vi "RT Main.vi"() -> ()   [LabVIEW 2018]
uses:
  <vilib>/rvi/interface/nirviOpenFPGA/nirviOpenFPGA.xnode
  <vilib>/rvi/interface/nirviMethod/nirviMethod.xnode
  <vilib>/FPGAPlugInAG/Dynamic/niLvFpga_Reset_Dynamic.vi
  <vilib>/FPGAPlugInAG/Dynamic/niLvFpga_Run_Dynamic.vi
  <vilib>/rvi/interface/nirviCloseFPGA/nirviCloseFPGA.xnode
  <vilib>/FPGAPlugInAG/Dynamic/niLvFpga_Close_Dynamic.vi
  <vilib>/FPGAPlugInAG/Dynamic/niLvFpga_Abort_Dynamic.vi
  <vilib>/rvi/interface/nirviReadWriteControl/nirviReadWriteControl.xnode
  NiFpgaLv.dll
  <vilib>/Utility/error.llb/Error Cluster From Error Code.vi
  <vilib>/rvi/interface/Simulation/niFpgaSimulationCallBeginRW.vi
  <vilib>/rvi/errors/niLvFpgaAdjustHostInterfaceError.vi
  <vilib>/ptbypt/NI_PtbyPt.lvlib
  <vilib>/addons/control/pid/NI_PID_pid.lvlib
  <vilib>/Analysis/NI_AALBase.lvlib
  <vilib>/Analysis/1siggen.llb/Ramp Pattern by Samples.vi
  FPGA Bitfiles/NVHLab_FPGATarget_MainFPGA_fVdYATQcYmw.lvbitx
  Main_FPGA.vi
  Controls/Output Range Brake.ctl
  Controls/Alarm1.ctl
  <vilib>/addons/control/pid/pid.llb/PID Output Rate Limiter (DBL).vi
  Controls/PID Gains.ctl
  Controls/Hydraulic1.ctl
  <vilib>/FPGAPlugInAG/cRIO-9082/niLvFpga_Open_cRIO-9082.vi
  <vilib>/rvi/interface/common/dynamic/niFpgaDynamicAddResources.vi
panel:
  out "Startwert Ramp H 2":dbl format="%#_3f"
  in  "stop 4":bool
  in  "stop 3":bool
  in  "stop 2":bool
  in  "Stop":bool
  in  "System Reset / ON":bool
  out "Alarms":T1
  in  "Alarme On":T2={"A 1"=TRUE, "A 2"=TRUE, "A 3"=TRUE, "A 4"=TRUE, "A 5"=TRUE, "A 6"=TRUE, "A 7"=TRUE, "A 8"=FALSE, "A 9"=TRUE, "A 10"=TRUE, "A 11"=TRUE, "A 12"=TRUE, "A 13"=TRUE, "A 14"=TRUE, "A 15"=TRUE, "A 16"=TRUE, "A 17"=TRUE, "A 18"=TRUE, "A 19"=TRUE, "A 20"=TRUE, "A 21"=TRUE, "A 22"=TRUE, "A 23"=TRUE, "A 24"=TRUE}
  in  "Master Alarm On":bool
  out "Master Alarm":bool
  in  "sample length LR":i32=100
  in  "sample length H":i32=100
  in  "Count (mSec) Normal LR":u32=10
  in  "Count (mSec) Ramp LR":u32=2
  in  "PID gains Brake L":T3={"proportional gain (Kc)"=0.3933188999071717, "integral gain (Kc*Ts/Ti)"=0.0018829701002687216, "derivative gain (Kc*Td/Ts)"=0.0} {"proportional gain (Kc)" format="%#_8g"; "integral gain (Kc*Ts/Ti)" format="%#_8g"}
  in  "PID gains Brake R":T3={"proportional gain (Kc)"=0.3933188999071717, "integral gain (Kc*Ts/Ti)"=0.0018829701002687216, "derivative gain (Kc*Td/Ts)"=0.0} {"proportional gain (Kc)" format="%#_8g"; "integral gain (Kc*Ts/Ti)" format="%#_8g"}
  in  "PID gains Brake H":T4={"proportional gain (Kc)"=5.0, "integral gain (Kc*Ts/Ti)"=0.1015625, "derivative gain (Kc*Td/Ts)"=0.0}
  in  "PID gains Speed Control":T4={"proportional gain (Kc)"=0.5, "integral gain (Kc*Ts/Ti)"=0.01171875, "derivative gain (Kc*Td/Ts)"=0.01171875}
  in  "sample length DM":i32=100
  in  "Count (mSec) Speed Control":u32=22
  in  "Count (mSec) H":u32=10
  in  "Output Range Brake R":T5={"Output high"=0.5, "Output low"=-0.5}
  in  "Output Range Brake L":T5={"Output high"=0.5, "Output low"=-0.5}
  in  "FeedFw_Ena":bool
  in  "Count (mSec) Ramp H":u32=2
  out "Mod6/Unit H":bool
  in  "output rate (EGU/min)":dbl=10000.0 format="%.2f"
  in  "Tq_Cal_H":cluster{"Gain_H":dbl, "Offset_H":dbl}={"Gain_H"=196.33, "Offset_H"=-10.8688} {"Offset_H" format="%#_13g"; "Gain_H" format="%#_13g"}
  in  "ACC_FeedFw":dbl
  in  "output range":T6={"output high"=10.0, "output low"=-3.0}
  in  "Speed_Ref_Cal_H":dbl
  in  "ESTOP":bool
  in  "Tq_Cal_L":cluster{"Gain":dbl, "Offset":dbl}={"Gain"=-175.0, "Offset"=-8.0} {"Offset" format="%#_13g"; "Gain" format="%#_13g"}
  in  "Tq_Cal_R":cluster{"Gain":dbl, "Offset":dbl}={"Gain"=-230.0, "Offset"=16.0} {"Offset" format="%#_13g"; "Gain" format="%#_13g"}
  in  "Spd_Cal_L":cluster{"Gain":dbl, "Offset":dbl}={"Gain"=298.85, "Offset"=0.0} {"Offset" format="%#_13g"; "Gain" format="%#_13g"}
  in  "Spd_Cal_R":cluster{"Gain":dbl, "Offset":dbl}={"Gain"=298.85, "Offset"=0.0} {"Offset" format="%#_13g"; "Gain" format="%#_13g"}
  in  "Spd_Cal_H":cluster{"Gain":dbl, "Offset":dbl}={"Gain"=800.0, "Offset"=100.0} {"Offset" format="%#_13g"; "Gain" format="%#_13g"}
  in  "milliseconds to wait Ramp LR":u32=10
  in  "type Ramp LR":u16(ring) items=["Linear", "Logarithmic"]
  out "Output Ramp LR":dbl format="%.2f"
  out "Output Speed Control":dbl
  in  "milliseconds to wait Speed Control":u32=10
  in  "type Speed Control":u16(ring) items=["Linear", "Logarithmic"]
  in  "milliseconds to wait Ramp H":u32=10
  in  "type Ramp H":u16(ring) items=["Linear", "Logarithmic"]
  out "Output Ramp H":dbl
  in  "Tab Control":enum32{"H", "L-R", "H-L-R", "System"}(tab)
  in  "Engine Speed/Torque H":bool
  in  "Torque Reference H":dbl(slide) scale=-1250.0..1250.0
  out "Torque with Transmission  H":dbl(knob) scale=-2000.0..2000.0
  out "Torque Back":dbl(knob) scale=-2000.0..2000.0
  out "Engine Speed Back":dbl(knob) scale=0.0..8000.0
  in  "Brake_H":bool
  in  "Direction H":bool=TRUE
  in  "Reset_H":bool
  in  "Control_H":bool
  in  "Speed_Ref_H":bool=TRUE caption="Torque_Ref_H"
  out "Report H":T7
  in  "Speed \nReferance H":dbl(slide) scale=0.0..8000.0
  out "Speed with Transmission H":dbl(knob) scale=0.0..12000.0
  in  "Transmisssion H":dbl=1.0
  in  "Start Ramp H":dbl=880.0
  in  "End Ramp H":dbl=4800.0
  in  "Time (Sec) Ramp H":i32=60
  out "Ramp H Activ":bool
  in  "Ramp H Stop":bool
  in  "Ramp H Down":bool
  in  "Ramp H Start":bool
  out "Ramp H  LED":bool
  out "Startwert Ramp H":dbl format="%#_3f"
  in  "Transmission with H":bool=TRUE
  out "Startwert Ramp LR":dbl format="%#_3f"
  out "Ramp LR  LED":bool
  in  "Transmission LR\nwith":bool=TRUE
  in  "Ramp LR Start":bool
  in  "Ramp LR Down":bool
  in  "Ramp LR Stop":bool
  out "Ramp LR active":bool
  in  "Time (Sec) Ramp LR":i32=60
  in  "End Ramp LR":dbl=4800.0
  in  "Start Ramp LR":dbl=880.0
  out "Speed_Diff":dbl(knob) scale=-30.0..30.0
  in  "Torque_Reference_LR":dbl(slide) caption="Torque \nReference" scale=-2000.0..2000.0
  in  "Engine Speed/moment LR":bool
  out "Torque with Transmission":dbl(knob) scale=-400.0..400.0
  out "Torque right":dbl(knob) scale=-2000.0..2000.0
  out "Torque left":dbl(knob) scale=-2000.0..2000.0
  out "Engine Speed right":dbl(knob) scale=0.0..3000.0
  out "Engine Speed left":dbl(knob) scale=0.0..3000.0
  in  "Brake_LR":bool
  in  "Direction\nBackwards":bool caption="Forward"
  in  "Reset_LR":bool
  in  "Control_LR":bool
  in  "Speed_Ref":bool=TRUE caption="Torque_Ref"
  out "Report L-R":T8
  in  "Speed_Reference_LR":dbl(slide) caption="Speed\n Reference" scale=0.0..3000.0
  out "Speed with Transmission":dbl(knob) scale=0.0..5000.0
  in  "Transmission LR":dbl=1.0
  out "L OUT":dbl
  out "R OUT":dbl
  in  "Loss Factor":dbl=1.0
  out "Speed With Trs HLR H 4":dbl caption="Torque With Transmission H"
  out "Speed With Trs HLR H 3":dbl caption="Speed With Transmission H"
  out "Speed With Trs HLR H 2":dbl caption="Torque With Transmission"
  out "Speed With Trs HLR H":dbl caption="Speed With Transmission"
  in  "Torque_Reference_LR 3":dbl(slide) caption="Torque \nReference H" scale=-2000.0..2000.0
  in  "Speed_Reference_LR 3":dbl(slide) caption="Speed\n Reference H" scale=0.0..3000.0
  in  "Torque_Reference_LR 2":dbl(slide) caption="Torque \nReference" scale=-2000.0..2000.0
  in  "Speed_Reference_LR 2":dbl(slide) caption="Speed\n Reference" scale=0.0..3000.0
  out "R OUT 2":dbl caption="R OUT"
  out "L OUT 2":dbl caption="L OUT"
  out "Speed_Diff 2":dbl(knob) scale=-30.0..30.0
  out "Engine Speed right HLR 2":dbl(knob) caption="Engine Speed Back" scale=0.0..3000.0
  out "Engine Speed right HLR":dbl(knob) caption="Engine Speed right" scale=0.0..3000.0
  out "Engine Speed left HLR":dbl(knob) caption="Engine Speed left" scale=0.0..3000.0
  in  "HLR LR Brake":T9={"Speed_Ref"=TRUE, "Control_HLR"=FALSE, "Reset_HLR"=FALSE, "Direction\nBackwards 2"=FALSE, "Brake_HLR"=FALSE} caption="HLR"
  in  "HLR H":T10={"Start Ramp H"=880.0, "End Ramp H"=4800.0, "Time (Sec) Ramp H"=60, "Ramp H Active"=FALSE, "Ramp H Stop"=FALSE, "Ramp H Down"=FALSE, "Ramp H Start"=FALSE, "Ramp H  LED 2"=FALSE, "Startwert Ramp H 2"=0.0} caption="H" {"Startwert Ramp H 2" format="%#_3f"}
  in  "HLR LR":T11={"H Time (Sec) Ramp LR"=60, "H Start Ramp LR"=880.0, "H End Ramp LR"=4800.0, "Startwert Ramp LR 2"=0.0, "H Ramp LR Start"=FALSE, "H Ramp LR Down"=FALSE, "H Ramp LR Stop"=FALSE, "Ramp LR  LED 2"=FALSE, "Ramp LR active"=FALSE, "Transmission LR\nwith"=TRUE} caption="LR" {"Startwert Ramp LR 2" format="%#_3f"}
  out "Report H-L-R":T12
  in  "Tab Control 2":enum32{"Petrol Engine", "Electric Engine"}(tab)
  in  "Mode_Section":u16(ring) items=["Idle", "N_Alfa", "N_T"]
  out "Ramp Cruise Control  LED":bool
  in  "Cruise Control Down":bool
  in  "Cruise Control Stop":bool
  out "Cruise Control Aktive":bool
  in  "Cruise Control Start":bool
  in  "PID Regler Speed Control\nWave Torque Reference":bool
  in  "Engine\nStart":bool
  in  "Pre Glow\nOn":bool
  in  "Ignition\nOn":bool
  in  "Fuel\nOn":bool
  out "Speed Control":u8(slide) scale=0.0..100.0
  in  "Speed Control Soll":dbl(slide) scale=0.0..100.0
  in  "Release Speed Control":bool
  in  "Clutch\nOpen":bool=TRUE
  out "Clutch":cluster{"Open":bool, "Closed":bool}
  in  "Time (Sec) Speed Control":i32=20
  in  "End Cruise Control":dbl=100.0
  in  "Start Cruise Control":dbl
  in  "Load Percent of Engine Speed":bool
  in  "Percent":dbl=0.5
  in  "Temperature Control \nRelease":bool
  in  "Temperature Control\nWait":bool
  in  "E-Acc_1":T13={"Gain"=1.0, "OffSet"=0.0}
  in  "E-Acc_2":T13={"Gain"=1.0, "OffSet"=0.0}
  out "High M":fxp<+/-,24,5> format="%#.2g"
  out "End Position \nDown M":bool
  out "End Position \nUp M":bool
  out "Up M":bool
  out "Down M":bool
  in  "Release High M":bool
  in  "Direction High M":bool
  in  "Release Engine Speed M":bool
  in  "Direction Engine Speed M":bool
  in  "Release Brake M":bool
  in  "Run Button":bool
  in  "Hydraulic Pump Control":dbl=11.0
  in  "Manual":bool
  in  "Up Button":bool
  in  "Down Button":bool
  in  "RPMK":dbl=300.0
  in  "Torque Engine":dbl
  in  "Hydraulic Clutch":dbl
  # "without"
  # "Left"
  # "Right"
  # "LR"
  # "without"
  # "Left"
  # "Right"
  # "H"
  # "System not Ready!"
  # "Closed"
  # "%"
  # "%"
  # "%"
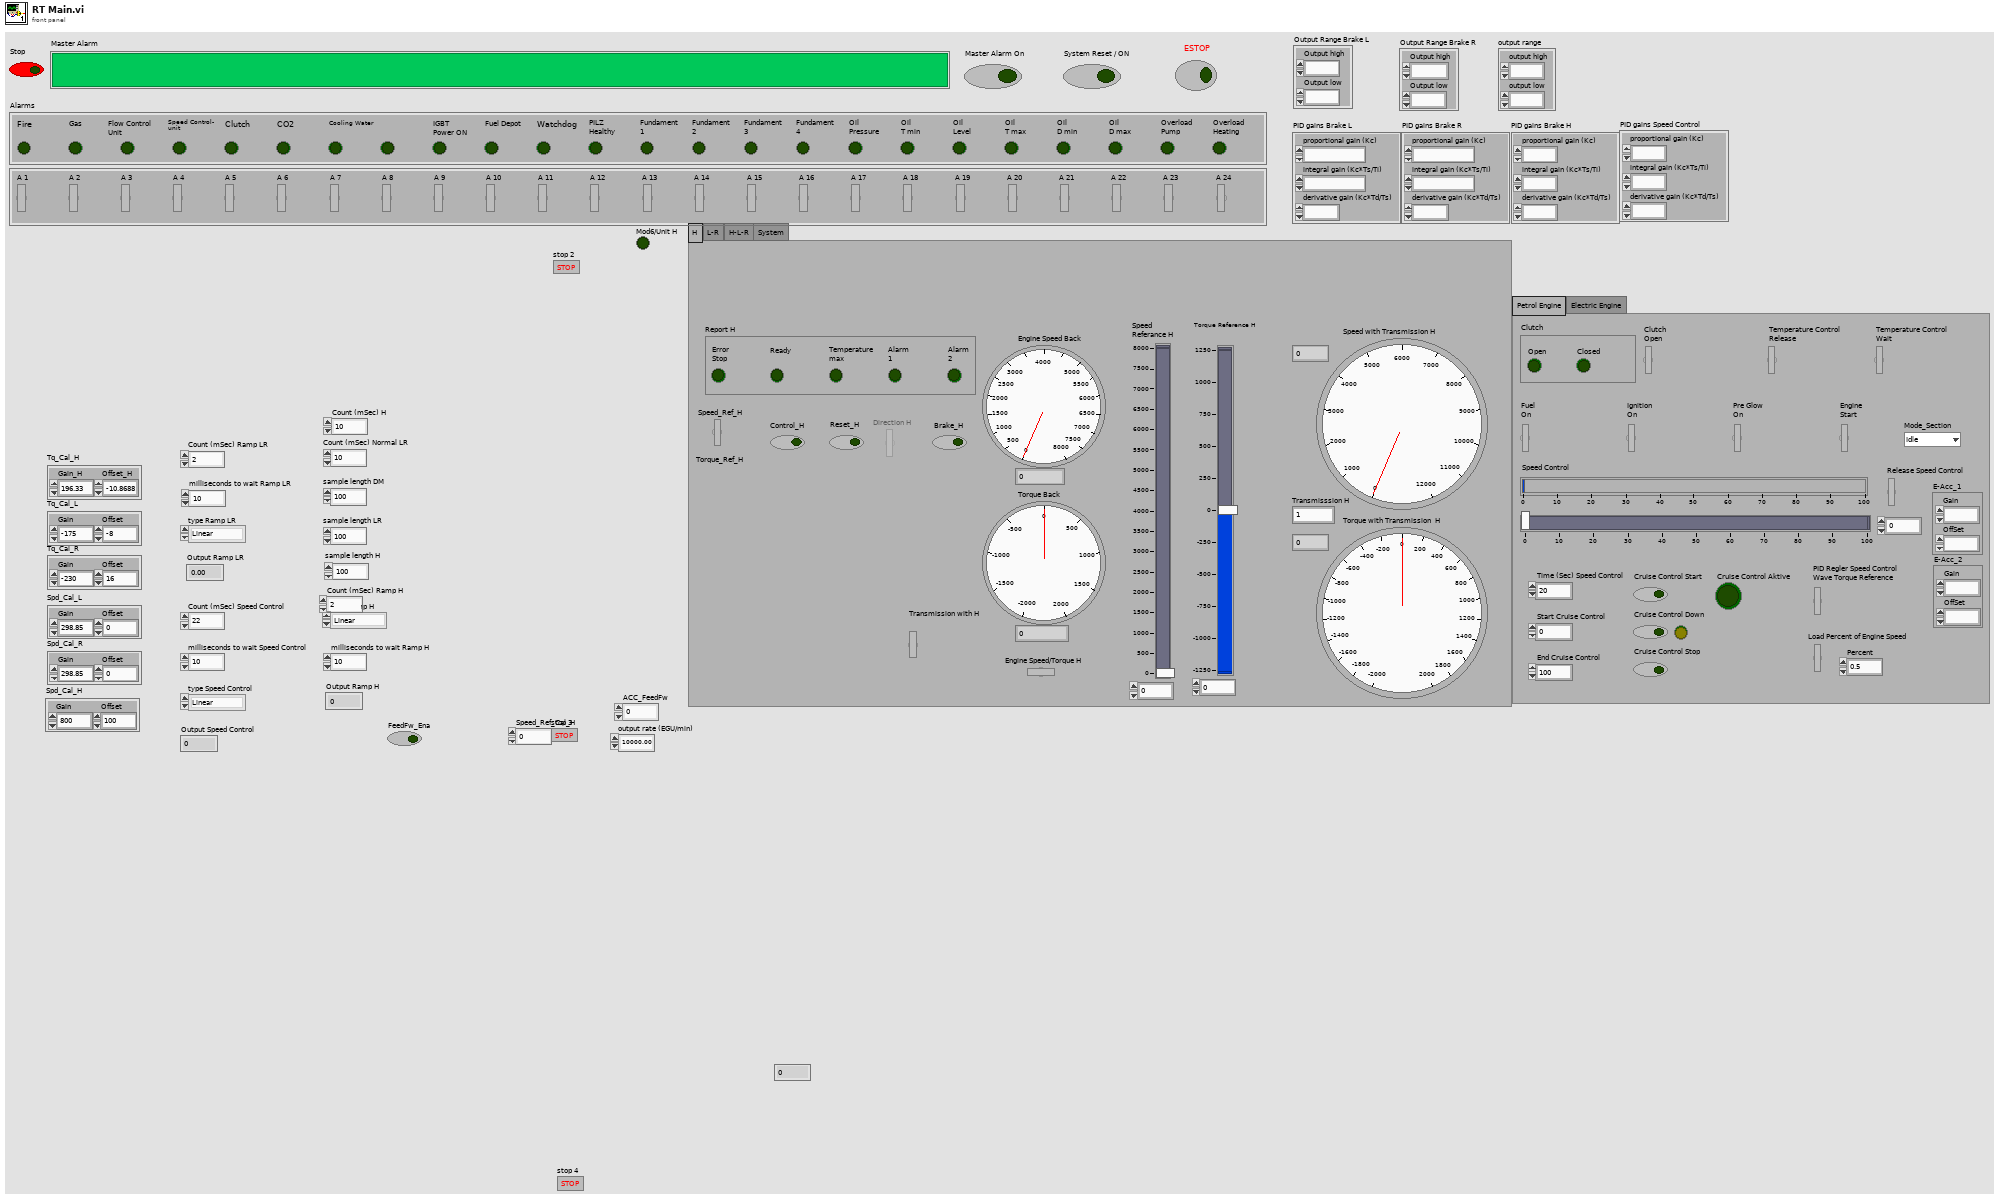
[diagram p1: front panel]
types:
  T1 = cluster{"Fire\n":bool, "Gas\n":bool, "Flow Control \nUnit":bool, "Speed Control-\nunit":bool, "Clutch\n":bool, "CO2\n":bool, "Cooling Water\n":bool, bool, "IGBT_ON":bool, "Fuel Depot\n":bool, "Watchdog\n":bool, "PILZ\nHealthy":bool, "Fundament\n1":bool, "Fundament\n2":bool, "Fundament\n3":bool, "Fundament\n4":bool, "Oil\nPressure":bool, "Oil\nT min":bool, "Oil\nLevel":bool, "Oil\nT max":bool, "Oil\nD min":bool, "Oil\nD max":bool, "Overload\nPump":bool, "Overload\nHeating":bool}
  T2 = typedef "Alarm1.ctl" = cluster{"A 1":bool, "A 2":bool, "A 3":bool, "A 4":bool, "A 5":bool, "A 6":bool, "A 7":bool, "A 8":bool, "A 9":bool, "A 10":bool, "A 11":bool, "A 12":bool, "A 13":bool, "A 14":bool, "A 15":bool, "A 16":bool, "A 17":bool, "A 18":bool, "A 19":bool, "A 20":bool, "A 21":bool, "A 22":bool, "A 23":bool, "A 24":bool}
  T3 = cluster{"proportional gain (Kc)":fxp<+/-,64,32>, "integral gain (Kc*Ts/Ti)":fxp<+/-,64,32>, "derivative gain (Kc*Td/Ts)":fxp<+/-,64,32>}
  T4 = cluster{"proportional gain (Kc)":fxp<+/-,16,8>, "integral gain (Kc*Ts/Ti)":fxp<+/-,16,8>, "derivative gain (Kc*Td/Ts)":fxp<+/-,16,8>}
  T5 = cluster{"Output high":fxp<+/-,64,32>, "Output low":fxp<+/-,64,32>}
  T6 = cluster{"output high":fxp<+/-,16,5>, "output low":fxp<+/-,16,5>}
  T7 = cluster{"Error\nStop":bool, "Ready\n":bool, "Temperature\nmax":bool, "Alarm\n1":bool, "Alarm\n2":bool}
  T8 = cluster{"Error\nStop":bool, "Ready\n":bool, "Temperature\nmax":bool, "Alarm\n1":bool, "Alarm\n2":bool, "Error\nStop":bool, "Ready\n":bool, "Temperature\nmax":bool, "Alarm\n1":bool, "Alarm\n2":bool}
  T9 = cluster{"Speed_Ref":bool, "Control_HLR":bool, "Reset_HLR":bool, "Direction\nBackwards 2":bool, "Brake_HLR":bool}
  T10 = cluster{"Start Ramp H":dbl, "End Ramp H":dbl, "Time (Sec) Ramp H":i32, "Ramp H Active":bool, "Ramp H Stop":bool, "Ramp H Down":bool, "Ramp H Start":bool, "Ramp H  LED 2":bool, "Startwert Ramp H 2":dbl}
  T11 = cluster{"H Time (Sec) Ramp LR":i32, "H Start Ramp LR":dbl, "H End Ramp LR":dbl, "Startwert Ramp LR 2":dbl, "H Ramp LR Start":bool, "H Ramp LR Down":bool, "H Ramp LR Stop":bool, "Ramp LR  LED 2":bool, "Ramp LR active":bool, "Transmission LR\nwith":bool}
  T12 = cluster{"Error\nStop":bool, "Ready\n":bool, "Temperature\nmax":bool, "Alarm\n1":bool, "Alarm\n2":bool, "Error\nStop":bool, "Ready\n":bool, "Temperature\nmax":bool, "Alarm\n1":bool, "Alarm\n2":bool, "H Error Stop\nStop 2":bool, "H Ready":bool, "H Temperature\nmax":bool, "H Alarm\n1":bool, "H Alarm2\n2":bool}
  T13 = cluster{"Gain":fxp<+/-,20,5>, "OffSet":fxp<+/-,20,5>}
  T14 = cluster{"Ramp Pattern":dbl[], "Ramp Type":u16, "Ramp Step":i32, "Ramp Start Cruise":dbl, "Ramp End  Cruise":dbl, "No of Ramps":i32, "Loop Time":u32, "LR Timer Done":bool, "LR Ramp On":bool, "Ramp Time Target":u32}
  T15 = cluster{"Ramp Pattern":dbl[], "Ramp Type":u16, "Ramp Step":i32, "Ramp Start H":dbl, "Ramp End  H":dbl, "No of Ramps":i32, "Loop Time":u32, "LR Timer Done":bool, "LR Ramp On":bool, "Ramp Time Target":u32}
  T16 = cluster{"FPGA VI Ref":refnum<k20>, "Ramp Pattern":dbl[], "Ramp Type":u16, "Ramp Step":i32, "Ramp Start LR":dbl, "Ramp End  LR":dbl, "No of Ramps":i32, "Loop Time":u32, "LR Timer Done":bool, "LR Ramp On":bool, "Ramp Time Target":u32}
  T17 = cluster{"System Reset / ON":bool, "Master Alarm On":bool, "Control_LR":bool, "Control_H":bool, "FeedFw_Ena":bool}
  T18 = typedef "Output Range Brake.ctl" = cluster{"Output Range Brake R":cluster{"Output high":fxp<+/-,64,32>, "Output low":fxp<+/-,64,32>}, "Output Range Brake L":cluster{"Output high":fxp<+/-,64,32>, "Output low":fxp<+/-,64,32>}, "output range":cluster{"output high":fxp<+/-,16,5>, "output low":fxp<+/-,16,5>}}
  T19 = typedef "PID Gains.ctl" = cluster{"PID gains Brake L":cluster{"proportional gain (Kc)":fxp<+/-,64,32>, "integral gain (Kc*Ts/Ti)":fxp<+/-,64,32>, "derivative gain (Kc*Td/Ts)":fxp<+/-,64,32>}, "PID gains Brake R":cluster{"proportional gain (Kc)":fxp<+/-,64,32>, "integral gain (Kc*Ts/Ti)":fxp<+/-,64,32>, "derivative gain (Kc*Td/Ts)":fxp<+/-,64,32>}, "PID gains Brake H":cluster{"proportional gain (Kc)":fxp<+/-,16,8>, "integral gain (Kc*Ts/Ti)":fxp<+/-,16,8>, "derivative gain (Kc*Td/Ts)":fxp<+/-,16,8>}, "PID gains Speed Control":cluster{"proportional gain (Kc)":fxp<+/-,16,8>, "integral gain (Kc*Ts/Ti)":fxp<+/-,16,8>, "derivative gain (Kc*Td/Ts)":fxp<+/-,16,8>}}
  T20 = typedef "Hydraulic1.ctl" = cluster{"Hydraulic Pump Control":dbl, "RPMK":dbl, "Down Button":bool, "Torque Engine":dbl, "Hydraulic Clutch":dbl, "Run Button":bool, "Up Button":bool}
  T21 = cluster{"Mod5/Alarm 1 Fire":bool, "Mod5/Alarm 2 Gas":bool, "Mod5/Alarm 3 Flow Control Unit":bool, "Mod5/Alarm 4 Speed Control":bool, "Mod5/Alarm 5 Clutch":bool, "Mod5/Alarm 6 CO2":bool, "Mod5/Alarm 7 Exhaust":bool, "Mod5/Alarm 8 Cooling Water":bool, "Mod5/Alarm 9 IGBT_ON":bool, "Mod5/Alarm 10 Fuel Depot":bool, "Mod5/Alarm 11 Watchdog":bool, "Mod5/Alarm 12 Spring Element":bool, "Mod5/Alarm 13 Fundament 1":bool, "Mod5/Alarm 14 Fundament 2":bool, "Mod5/Alarm 15 Fundament 3":bool, "Mod5/Alarm 16 Fundament 4":bool, "Mod6/Alarm 17 Oil Pressure Difference":bool, "Mod6/Alarm 19 min Oil Pressure":bool, "Mod6/Alarm 18 Oil Level":bool, "Mod6/Alarm 20 max Oil Temperature":bool, "Mod6/Alarm 21 min Oil Pressure":bool, "Mod6/Alarm 22 max Oil Pressure":bool, "Mod6/Alarm 23 Overload Warning Oil Pump":bool, "Mod6/Alarm 24 Overload Warning Oil Heating":bool}
  T22 = cluster{"Mod5/Error Brake L":bool, "Mod5/Ready Brake L":bool, "Mod5/Temperature Brake L":bool, "Mod5/Alarm 1 Brake L":bool, "Mod5/Alarm 2 Brake L":bool, "Mod5/Error Brake R":bool, "Mod5/Ready Brake R":bool, "Mod5/Temperature Brake R":bool, "Mod5/Alarm 1 Brake R":bool, "Mod5/Alarm 2 Brake R":bool}
  T23 = cluster{"Mod6/Error Brake back":bool, "Mod6/Ready Brake back":bool, "Mod6/Temperature Brake back":bool, "Mod6/Alarm 1 Brake back":bool, "Mod6/Alarm 2 Brake back":bool}
  T24 = cluster{"Mod6/Clutch open":bool, "Mod6/Clutch closed":bool}
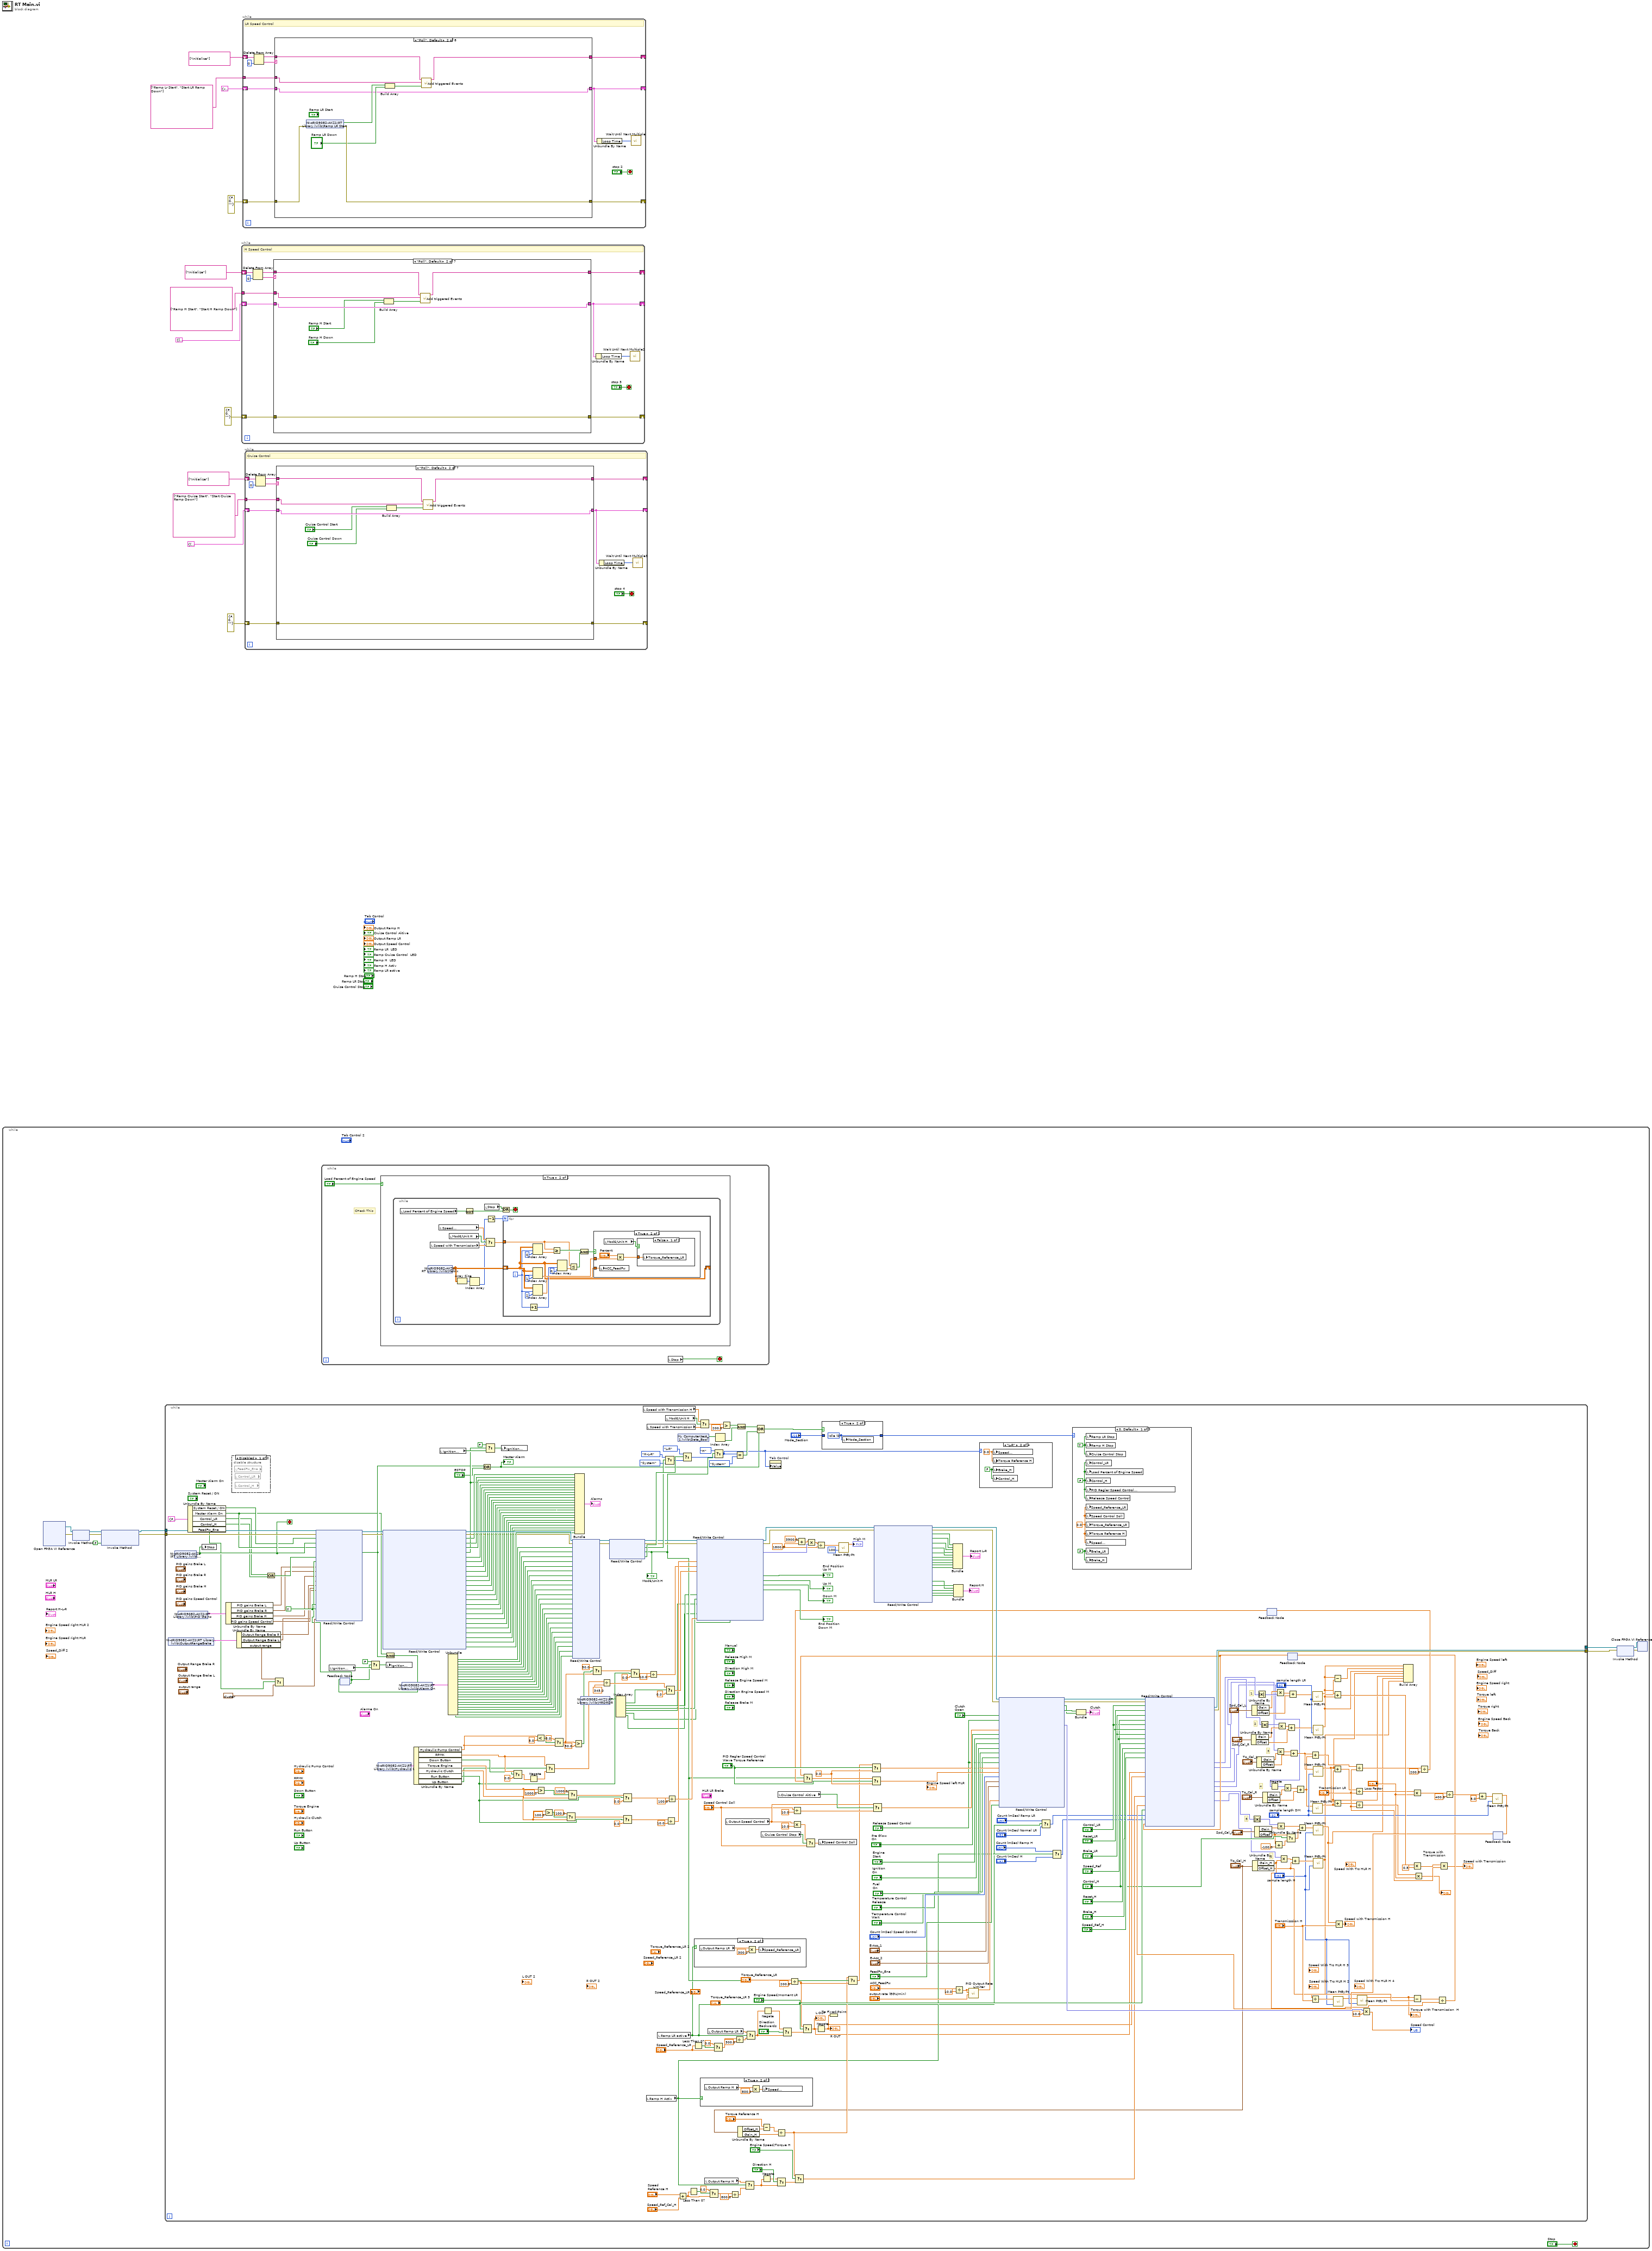
[diagram p0: block diagram]
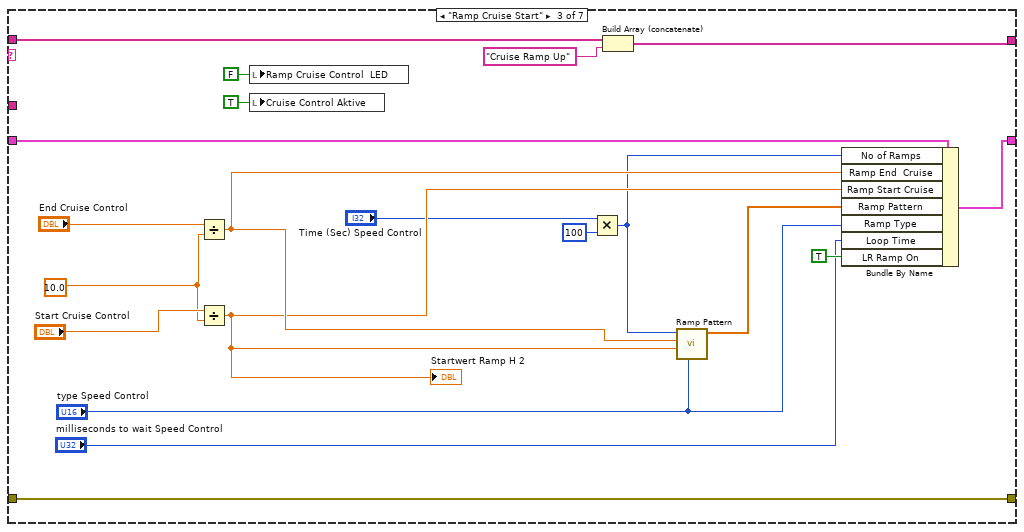
[diagram p3: hidden frame]
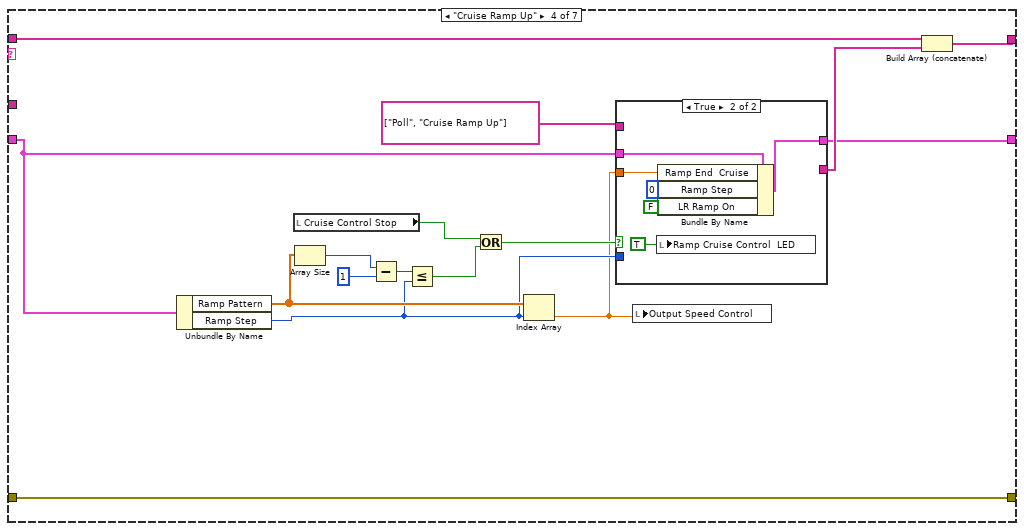
[diagram p4: hidden frame]
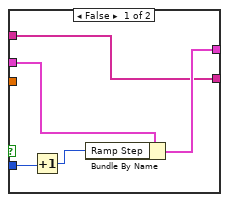
[diagram p5: hidden frame]
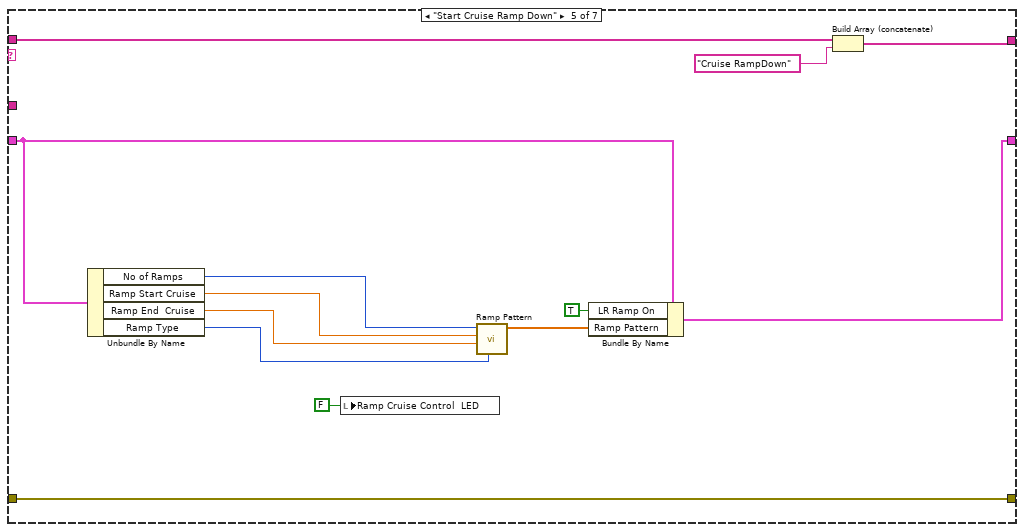
[diagram p6: hidden frame]
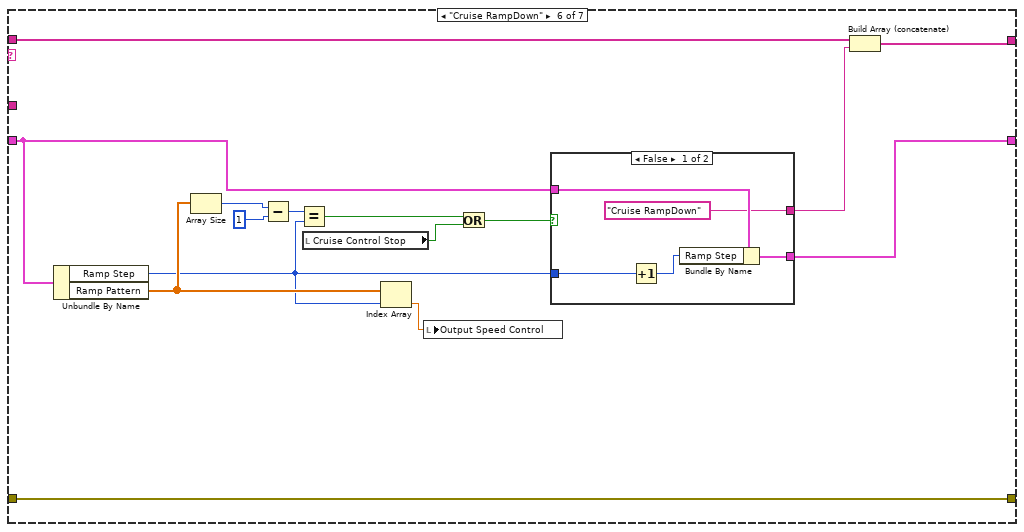
[diagram p7: hidden frame]
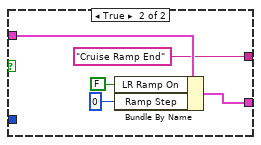
[diagram p8: hidden frame]
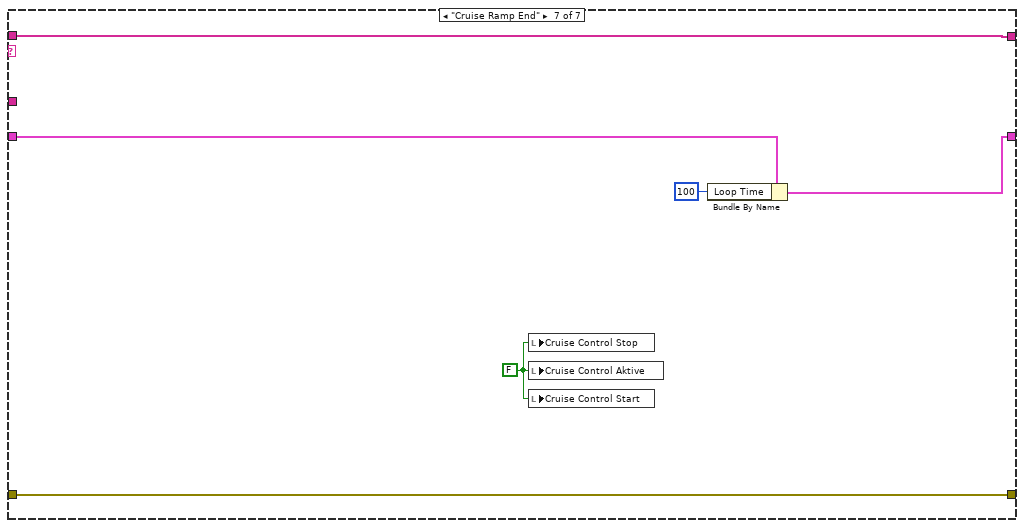
[diagram p9: hidden frame]
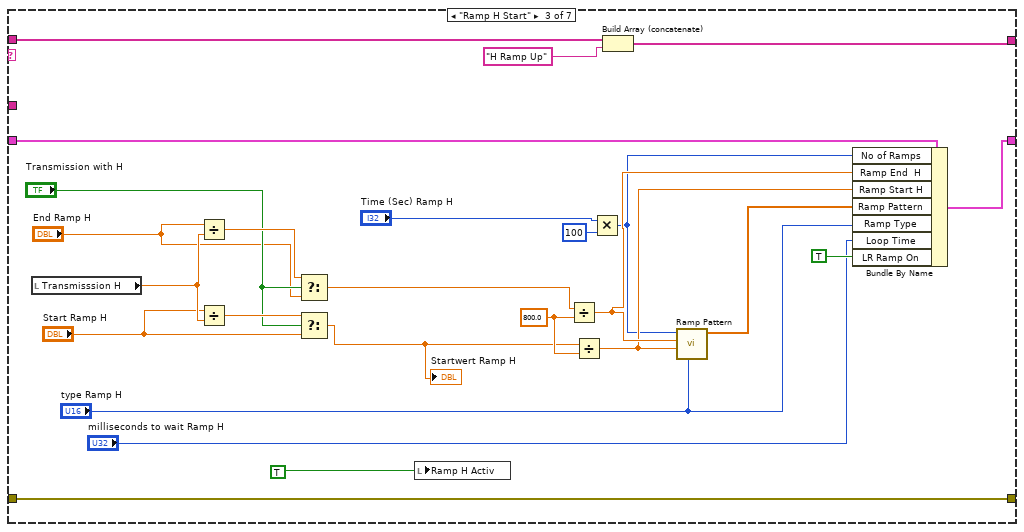
[diagram p11: hidden frame]
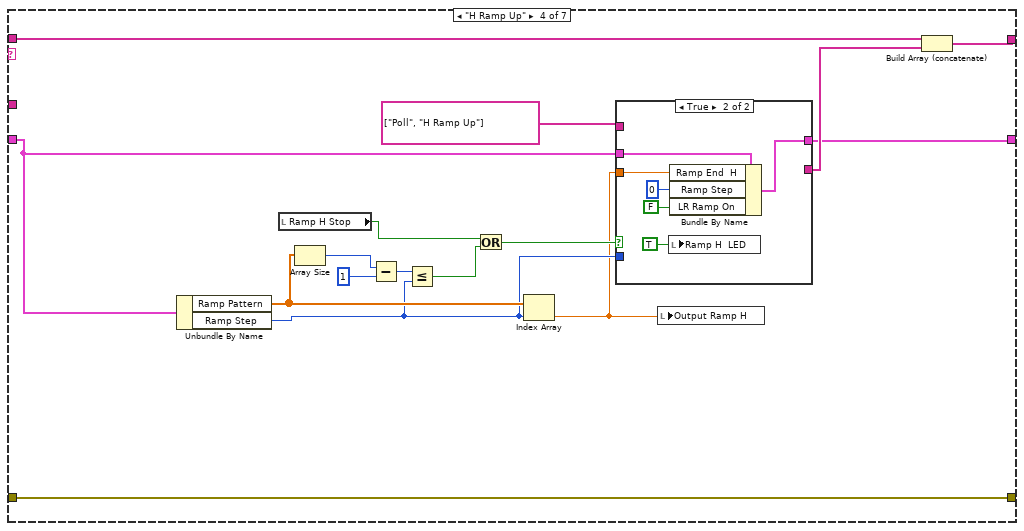
[diagram p12: hidden frame]
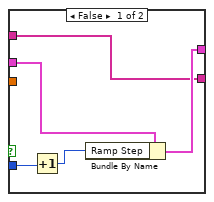
[diagram p13: hidden frame]
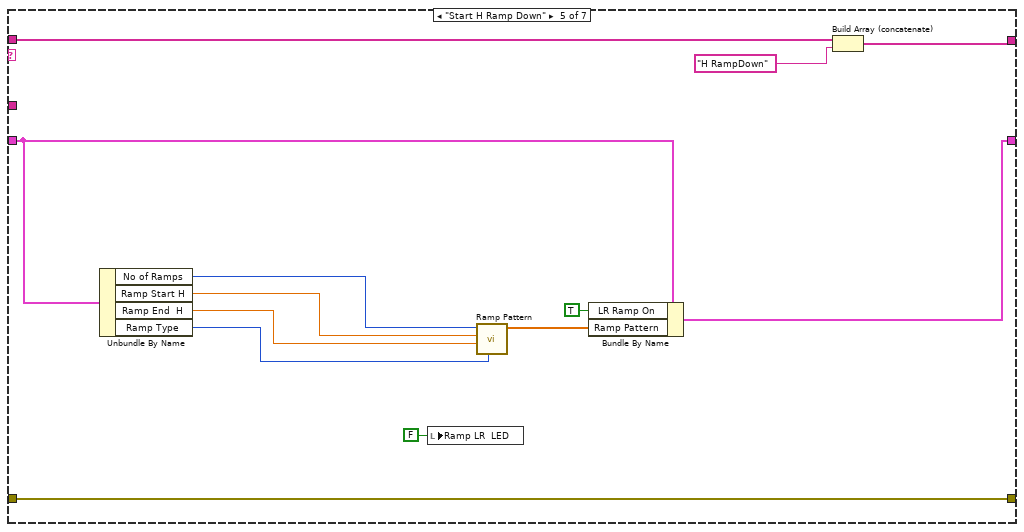
[diagram p14: hidden frame]
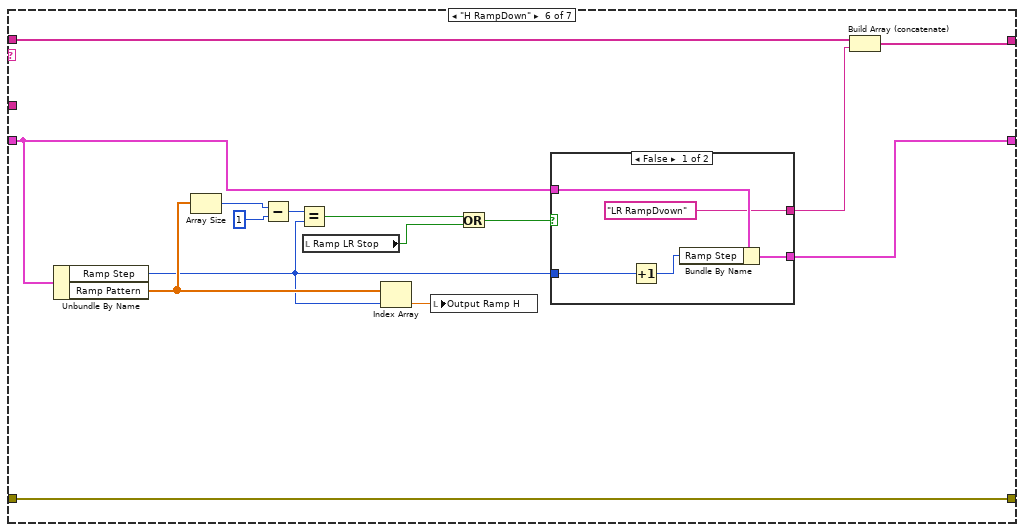
[diagram p15: hidden frame]
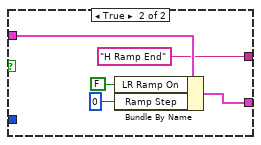
[diagram p16: hidden frame]
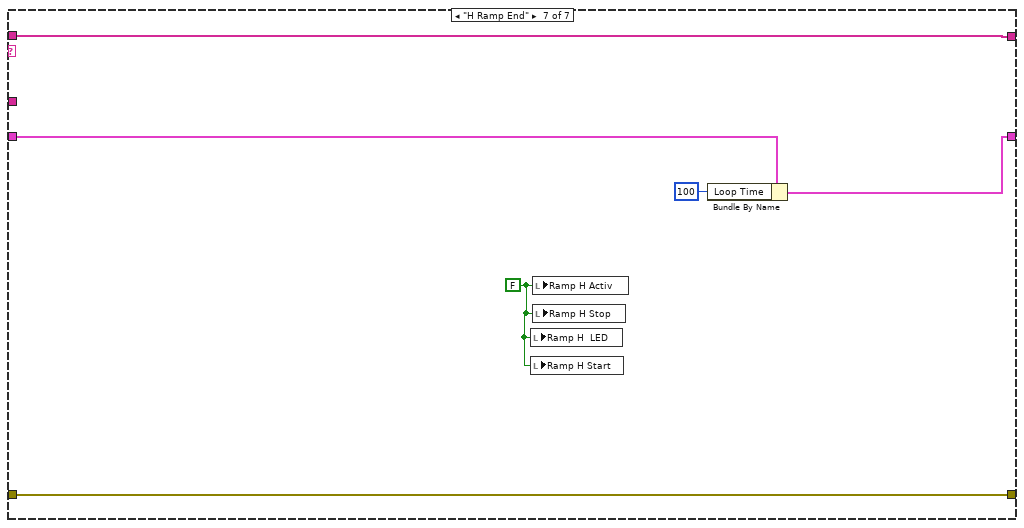
[diagram p17: hidden frame]
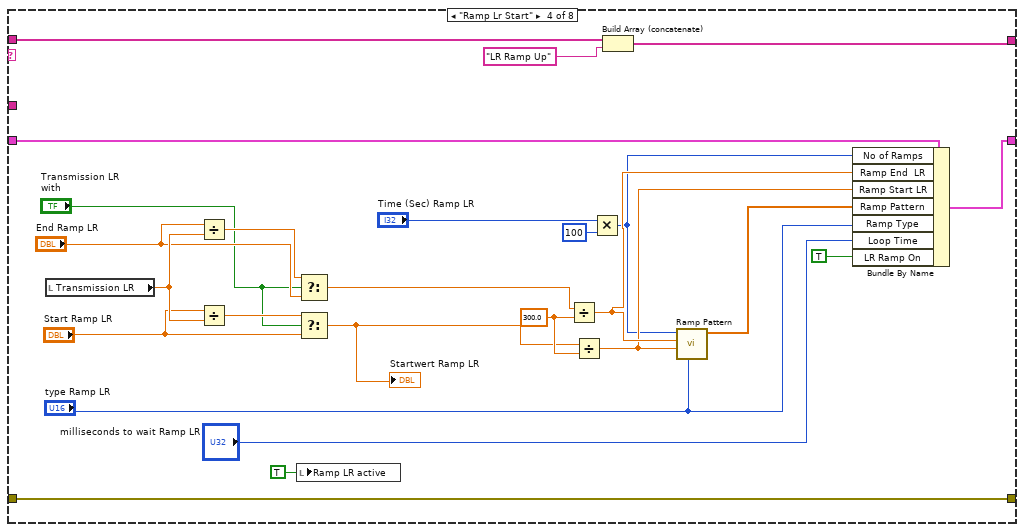
[diagram p20: hidden frame]
diagram:
  n1 = while {
    stop <- "Stop" stop-if-true
    n2 = xnode "Open FPGA VI Reference"() -> ("FPGA VI Reference Out"=w20:refnum<k20>, "error out"=w19:errorcluster)  [unwired: 2 in]
    n3 = xnode "Invoke Method"("FPGA VI Reference In"=w20, "error in"=w19) -> ("FPGA VI Reference Out"=w18:refnum<k20>, "error out"=w17:errorcluster)
    n4 = xnode "Invoke Method"("FPGA VI Reference In"=w18, "error in"=w17, "Wait Until Done (F)"=FALSE) -> ("FPGA VI Reference Out"=w13:refnum<k20>, "error out"=w24:errorcluster)
    n5 = while {
      tunnel: w13 -> [w439]
      tunnel: w24 -> [w438]
      tunnel: [w279] -> w23
      tunnel: [w308] -> w21
      stop <- w85 stop-if-true
      w220 = TRUE
      w261 = 0.0 ("f")
      w344 = 1800.0 ("y")
      # "6"
      # "5"
      # "4"
      # "3"
      # "2"
      # "1"
      n6 = shared-variable "NI-cRIO9082-AKZ1\\RT Library.lvlib\\OutputRangeBrake"() -> (w81:T18)  [unwired: 1 in, 1 out]
      n7 = shared-variable "NI-cRIO9082-AKZ1\\RT Library.lvlib\\Stop"() -> (w85:bool)  [unwired: 1 in, 1 out]
      n8 = shared-variable "NI-cRIO9082-AKZ1\\RT Library.lvlib\\PID Gains"() -> (w86:T19)  [unwired: 1 in, 1 out]
      n9 = Unbundle By Name(T17 {"System Reset / ON"=FALSE, "Master Alarm On"=FALSE, "Control_LR"=FALSE, "Control_H"=FALSE, "FeedFw_Ena"=FALSE}) -> ("System Reset / ON"=w79:bool, "Master Alarm On"=w78:bool, "Control_LR"=w77:bool, "Control_H"=w76:bool, "FeedFw_Ena"=w75:bool)
      n10 = local write "Stop"(w85) -> ()
      n11 = Unbundle By Name(w86) -> ("PID gains Brake L"=w90:T3, "PID gains Brake R"=w89:T3, "PID gains Brake H"=w88:T4, "PID gains Speed Control"=w87:T4)
      n12 = disable-structure shown="Disabled" {
        frame Disabled {
          n13 = local read "FeedFw_Ena"() -> ()  [unwired: 1 out]
          n14 = local read "Control_LR"() -> ()  [unwired: 1 out]
          n15 = local read "Control_H"() -> ()  [unwired: 1 out]
        }
        frame Enabled {
        }
      }
      n16 = Unbundle By Name(w81) -> ("Output Range Brake R"=w84:T5, "Output Range Brake L"=w83:T5, "output range"=w82:T6)
      n17 = Or(x=w77, y=w76) -> (x .or. y?=w288:bool)
      n18 = Select(t=w82, s=w75, f=T6 {"output high"=10.0, "output low"=0.0} ("output range")) -> (s? t:f=w176:T6)
      n19 = local read "Ignition\nOn"() -> (w238:bool)
      n20 = feedback #1() -> (w151:bool)  [unwired: 1 in]
      n21 = xnode "Read/Write Control"("FPGA VI Reference In"=w439, "error in"=w438, "Mod3/System Reset/ON"=w79, "STOP"=w85, "Alarm ON"=w78, "Mod3/Flashing light"=w288, "Mod3/Horn"=w151, "PID gains Brake L"=w90, "PID gains Brake R"=w89, "PID gains Brake H"=w88, "PID gains"=w87, "Output Range Brake R"=w84, "Output Range Brake L"=w83, "PID Out LR"=w220, "PID Out H"=w220, "output range"=w176) -> ("FPGA VI Reference Out"=w437:refnum<k20>, "error out"=w353:errorcluster, "Alarm"=w150:bool)  [unwired: 3 out]
      n22 = Select(t=FALSE, s=w151, f=w238) -> (s? t:f=w240:bool)
      n23 = shared-variable "NI-cRIO9082-AKZ1\\RT Library.lvlib\\Hydraulic 1"() -> (w92:T20)  [unwired: 1 in, 1 out]
      n24 = xnode "Read/Write Control"("FPGA VI Reference In"=w437, "error in"=w353) -> ("FPGA VI Reference Out"=w436:refnum<k20>, "error out"=w314:errorcluster, "Mod5/Alarm 1 Fire"=w435:bool, "Mod5/Alarm 2 Gas"=w434:bool, "Mod5/Alarm 3 Flow Control Unit"=w432:bool, "Mod5/Alarm 4 Speed Control"=w232:bool, "Mod5/Alarm 5 Clutch"=w431:bool, "Mod5/Alarm 6 CO2"=w430:bool, "Mod5/Alarm 7 Exhaust"=w215:bool, "Mod5/Alarm 8 Cooling Water"=w429:bool, "Mod5/Alarm 9 IGBT_ON"=w428:bool, "Mod5/Alarm 10 Fuel Depot"=w427:bool, "Mod5/Alarm 11 Watchdog"=w426:bool, "Mod5/Alarm 12 Spring Element"=w425:bool, "Mod5/Alarm 13 Fundament 1"=w424:bool, "Mod5/Alarm 14 Fundament 2"=w423:bool, "Mod5/Alarm 15 Fundament 3"=w422:bool, "Mod5/Alarm 16 Fundament 4"=w421:bool, "Mod6/Alarm 17 Oil Pressure Difference"=w420:bool, "Mod6/Alarm 19 min Oil Pressure"=w419:bool, "Mod6/Alarm 18 Oil Level"=w418:bool, "Mod6/Alarm 20 max Oil Temperature"=w417:bool, "Mod6/Alarm 21 min Oil Pressure"=w416:bool, "Mod6/Alarm 22 max Oil Pressure"=w415:bool, "Mod6/Alarm 23 Overload Warning Oil Pump"=w414:bool, "Mod6/Alarm 24 Overload Warning Oil Heating"=w413:bool)
      n25 = And(x=w78, y=w150) -> (x .and. y?=w363:bool)
      n26 = feedback-in #1(w363) -> ()
      n27 = local write "Ignition\nOn"(w240) -> ()
      n28 = shared-variable "NI-cRIO9082-AKZ1\\RT Library.lvlib\\Alarm On"() -> (w91:T2)  [unwired: 1 in, 1 out]
      n29 = Unbundle By Name(w92) -> ("Hydraulic Pump Control"=w99:dbl, "RPMK"=w98:dbl, "Down Button"=w97:bool, "Torque Engine"=w96:dbl, "Hydraulic Clutch"=w95:dbl, "Run Button"=w94:bool, "Up Button"=w93:bool)
      n30 = local read "Ignition\nOn"() -> (w235:bool)
      n31 = Unbundle(w91) -> ("A 1"=w411:bool, "A 2"=w410:bool, "A 3"=w409:bool, "A 4"=w408:bool, "A 5"=w407:bool, "A 6"=w406:bool, "A 7"=w405:bool, "A 8"=w404:bool, "A 9"=w403:bool, "A 10"=w402:bool, "A 11"=w401:bool, "A 12"=w400:bool, "A 13"=w399:bool, "A 14"=w398:bool, "A 15"=w397:bool, "A 16"=w396:bool, "A 17"=w395:bool, "A 18"=w394:bool, "A 19"=w393:bool, "A 20"=w392:bool, "A 21"=w391:bool, "A 22"=w390:bool, "A 23"=w389:bool, "A 24"=w388:bool)
      n32 = Or(x=w150, y="ESTOP") -> (x .or. y?=w149:bool)
      "Master Alarm" <- w149
      n33 = Select(t=FALSE, s=w232, f=w235) -> (s? t:f=w233:bool)
      n34 = local write "Ignition\nOn"(w233) -> ()
      n35 = Select(t=w98, s=w97, f=0.0) -> (s? t:f=w338:dbl)
      n36 = Negate(x=w338) -> (-x=w337:dbl)
      n37 = Less?(x=w99, y=5.0) -> (x < y?=w276:bool)
      n38 = Greater?(x=w96, y=1000.0) -> (0:w321:bool)
      n39 = Greater?(x=w95, y=100.0) -> (0:w285:bool)
      n40 = Select(t=w98, s=w93, f=w337) -> (s? t:f=w336:dbl)
      n41 = Select(t=5.0, s=w276, f=w99) -> (s? t:f=w274:dbl)
      n42 = Select(t=100.0, s=w285, f=w95) -> (s? t:f=w283:dbl)
      n43 = Select(t=1000.0, s=w321, f=w96) -> (s? t:f=w318:dbl)
      n44 = xnode "Read/Write Control"("FPGA VI Reference In"=w436, "error in"=w314, "Alarm 1 ON"=w411, "Alarm 2 ON"=w410, "Alarm 3 ON"=w409, "Alarm 4 ON"=w408, "Alarm 5 ON"=w407, "Alarm 6 ON"=w406, "Alarm 7 ON"=w405, "Alarm 8 ON"=w404, "Alarm 9 ON"=w403, "Alarm 10 ON"=w402, "Alarm 11 ON"=w401, "Alarm 12 ON"=w400, "Alarm 13 ON"=w399, "Alarm 14 ON"=w398, "Alarm 15 ON"=w397, "Alarm 16 ON"=w396, "Alarm 17 ON"=w395, "Alarm 18 ON"=w394, "Alarm 19 ON"=w393, "Alarm 20 ON"=w392, "Alarm 21 ON"=w391, "Alarm 22 ON"=w390, "Alarm 23 ON"=w389, "Alarm 24 ON"=w388) -> ("FPGA VI Reference Out"=w412:refnum<k20>, "error out"=w313:errorcluster)
      n45 = Greater?(x=w274, y=50.0) -> (0:w331:bool)
      n46 = Bundle("Mod5/Alarm 1 Fire"=w435, "Mod5/Alarm 2 Gas"=w434, "Mod5/Alarm 3 Flow Control Unit"=w432, "Mod5/Alarm 4 Speed Control"=w232, "Mod5/Alarm 5 Clutch"=w431, "Mod5/Alarm 6 CO2"=w430, "Mod5/Alarm 7 Exhaust"=w215, "Mod5/Alarm 8 Cooling Water"=w429, "Mod5/Alarm 9 IGBT_ON"=w428, "Mod5/Alarm 10 Fuel Depot"=w427, "Mod5/Alarm 11 Watchdog"=w426, "Mod5/Alarm 12 Spring Element"=w425, "Mod5/Alarm 13 Fundament 1"=w424, "Mod5/Alarm 14 Fundament 2"=w423, "Mod5/Alarm 15 Fundament 3"=w422, "Mod5/Alarm 16 Fundament 4"=w421, "Mod6/Alarm 17 Oil Pressure Difference"=w420, "Mod6/Alarm 19 min Oil Pressure"=w419, "Mod6/Alarm 18 Oil Level"=w418, "Mod6/Alarm 20 max Oil Temperature"=w417, "Mod6/Alarm 21 min Oil Pressure"=w416, "Mod6/Alarm 22 max Oil Pressure"=w415, "Mod6/Alarm 23 Overload Warning Oil Pump"=w414, "Mod6/Alarm 24 Overload Warning Oil Heating"=w413) -> (→"Alarms":T21)  [unwired: 1 in]
      n47 = shared-variable "NI-cRIO9082-AKZ1\\RT Library.lvlib\\MRDRDR"() -> (w100:bool[])  [unwired: 1 in, 1 out]
      n48 = Select(t=50.0, s=w331, f=w274) -> (s? t:f=w286:dbl)
      n49 = Divide(x=w336, y=345.0) -> (x/y=w334:dbl)
      n50 = xnode "Read/Write Control"("FPGA VI Reference In"=w412, "error in"=w313) -> ("FPGA VI Reference Out"=w328:refnum<k20>, "error out"=w312:errorcluster, "Mod6/Unit H-L-R"=w385:bool, "Mod6/Unit H"=w205:bool, "Mod6/Unit L-R"=w387:bool)
      "Mod6/Unit H" <- w205
      n51 = Index Array(array=w100) -> (element #1=w106:bool, element #2=w105:bool, element #3=w104:bool, element #4=w103:bool, element #5=w102:bool, element #6=w101:bool)  [unwired: 6 in]
      n52 = Select(t=w318, s=w94, f=0.0) -> (s? t:f=w317:dbl)
      n53 = Select(t=w283, s=w94, f=0.0) -> (s? t:f=w282:dbl)
      n54 = Select(t=w286, s=w94, f=0.0) -> (s? t:f=w340:dbl)
      n55 = local read "Speed with Transmission H"() -> (w163:dbl)
      n56 = local read "Ramp H Activ"() -> (w194:bool)
      n57 = local read "Speed with Transmission"() -> (w162:dbl)
      n58 = Divide(x=w340, y=10.0) -> (x/y=w270:dbl)
      n59 = local read "Ramp LR active"() -> (w122:bool)
      n60 = Select(t=enum32{"H", "L-R", "H-L-R", "System"}."H-L-R" ("Tab Control"), s=w385, f=enum32{"H", "L-R", "H-L-R", "System"}."System" ("Tab Control")) -> (s? t:f=w386:enum32{"H", "L-R", "H-L-R", "System"})
      n61 = Select(t=w334, s=w106, f=0.0) -> (s? t:f=w329:dbl)
      n62 = local read "Mod6/Unit H"() -> (w164:bool)
      n63 = Divide(x=w282, y=10.0) -> (x/y=w280:dbl)
      n64 = Divide(x=w317, y=100.0) -> (x/y=w315:dbl)
      n65 = shared-variable "My Computer\\test_1.lvlib\\Data_Bool"() -> (w195:bool[])  [unwired: 1 in, 1 out]
      n66 = Add(x="Speed \nReferance H", y="Speed_Ref_Cal_H") -> (x+y=w173:dbl)
      n67 = Select(t=enum32{"H", "L-R", "H-L-R", "System"}."L-R" ("Tab Control"), s=w387, f=w386) -> (s? t:f=w153:enum32{"H", "L-R", "H-L-R", "System"})
      n68 = Less Than 0?(x=w173) -> (x < 0?=w301:bool)
      n69 = Less Than 0?(x="Speed_Reference_LR") -> (x < 0?=w307:bool)
      n70 = case shown="True" w122 {
        frame False {
        }
        frame True {
          n71 = local read "Output Ramp LR"() -> (w441:dbl)
          n72 = Multiply(x=w441, y=300.0 ("Faktor RL")) -> (x*y=w440:dbl)
          n73 = local write "Speed_Reference_LR"(w440) -> ()
        }
      }
      n74 = xnode "Read/Write Control"("FPGA VI Reference In"=w328, "error in"=w312, "Mod7/Hydraulic clutch Set point"=w280, "Mod7/Hydraulic pump actuator Soll"=w270, "Mod7/Up M Set point"=w329, "Mod4/Release Up M"=w105, "Mod4/Richtung Up M"=w104, "Mod4/Release Engine Speed M"=w103, "Mod4/Richtung Engine Speed M"=w102, "Mod4/Release Brake M"=w101, "Mod7/Torque M Set point"=w315) -> ("FPGA VI Reference Out"=w225:refnum<k20>, "error out"=w311:errorcluster, "Mod8/Up M"=w346:fxp<+/-,24,5>, "Mod6/End Position UP M"=→"End Position \nUp M":bool, "Mod6/UP M"=→"Up M":bool, "Mod6/DOWN M"=→"Down M":bool, "Mod6/End Position DOWN M"=→"End Position \nDown M":bool)  [unwired: 2 out]
      n75 = Select(t=w163, s=w164, f=w162) -> (s? t:f=w161:dbl)
      n76 = case shown="True" w194 {
        frame False {
        }
        frame True {
          n77 = local read "Output Ramp H"() -> (w451:dbl)
          n78 = Multiply(x=w451, y=800.0) -> (x*y=w450:dbl)
          n79 = local write "Speed \nReferance H"(w450) -> ()
        }
      }
      n80 = local read "Output Ramp H"() -> (w219:dbl)
      n81 = local read "Output Ramp LR"() -> (w226:dbl)
      n82 = Select(t=0.0, s=w301, f=w173) -> (s? t:f=w299:dbl)
      n83 = Select(t=0.0, s=w307, f="Speed_Reference_LR") -> (s? t:f=w264:dbl)
      n84 = Select(t=enum32{"H", "L-R", "H-L-R", "System"}."H" ("Tab Control"), s=w205, f=w153) -> (s? t:f=w157:enum32{"H", "L-R", "H-L-R", "System"})
      n85 = Index Array(array=w195) -> (element=w191:bool)  [unwired: 1 in]
      n86 = Greater?(x=w161, y=200.0) -> (0:w192:bool)
      n87 = local read "Output Speed Control"() -> (w252:dbl)
      n88 = Divide(x=w299, y=800.0) -> (x/y=w117:dbl)
      n89 = Divide(x=w264, y=300.0 ("Faktor RL")) -> (x/y=w269:dbl)
      n90 = Equal?(x=w157, y=enum32{"H", "L-R", "H-L-R", "System"}."System" ("s? t:f")) -> (x = y?=w159:bool)
      n91 = And(x=w192, y=w191) -> (x .and. y?=w160:bool)
      n92 = Unbundle By Name("Tq_Cal_H") -> ("Offset_H"=w189:dbl, "Gain_H"=w188:dbl)
      n93 = Select(t=w219, s=w194, f=w117) -> (s? t:f=w116:dbl)
      n94 = Select(t=w226, s=w122, f=w269) -> (s? t:f=w230:dbl)
      n95 = Compound Arithmetic op=OR(w160, w149, w159) -> (w147:bool)
      n96 = local read "Cruise Control Stop"() -> (w255:bool)
      n97 = Subtract(x="Torque Reference H", y=w189) -> (x-y=w187:dbl)
      n98 = Negate(x=w116) -> (-x=w297:dbl)
      n99 = Negate(x=w230) -> (-x=w367:dbl)
      n100 = property on="Tab Control" class="TabCtl (strict)"("Value"=w157) -> ()  [unwired: 2 in, 2 out]
      n101 = Divide(x=w187, y=w188) -> (x/y=w204:dbl)
      n102 = Select(t=w297, s="Direction H", f=w116) -> (s? t:f=w115:dbl)
      n103 = local read "Cruise Control Aktive"() -> (w256:bool)
      n104 = Select(t=w367, s="Direction\nBackwards", f=w230) -> (s? t:f=w229:dbl)
      n105 = Divide(x="Torque_Reference_LR", y=200.0) -> (x/y=w207:dbl)
      n106 = Divide(x="Speed Control Soll", y=10.0) -> (x/y=w251:dbl)
      n107 = Multiply(x=w252, y=10.0) -> (x*y=w253:dbl)
      n108 = Select(t=w204, s="Engine Speed/Torque H", f=w115) -> (s? t:f=w211:dbl)
      n109 = Add(x=3900.0, y=w344) -> (x+y=w347:dbl)
      n110 = Select(t=w207, s="Engine Speed/moment LR", f=w229) -> (s? t:f=w124:dbl)
      "L OUT" <- w124
      n111 = Select(t=w253, s=w255, f="Speed Control Soll") -> (s? t:f=w254:dbl)
      n112 = Multiply(x=w347, y=w346) -> (x*y=w345:dbl)
      n113 = Divide(x=w345, y=w344) -> (x/y=w342:dbl)
      n114 = Negate(x=w124) -> (-x=w123:dbl)
      "R OUT" <- w123
      n115 = local write "Speed Control Soll"(w254) -> ()
      n116 = case shown="True" w147 {
        tunnel: [w443 w444] -> w146
        tunnel: "Mode_Section" -> [w443 _]
        frame False {
        }
        frame True {
          w444 = u16 0 items=["Idle", "N_Alfa", "N_T"] ("Mode_Section")
          n117 = local write "Mode_Section"(w444) -> ()
        }
      }
      n118 = To Fixed-Point(number=w123) -> ()  [unwired: 1 in, 1 out]
      n119 = call <vilib>:"Mean PtByPt.vi"("x"=w342, "sample length"=100) -> ("mean"=→"High M":dbl)  [unwired: 2 in, 1 out]
      n120 = Select(t=w204, s=w205, f=w207) -> (s? t:f=w206:dbl)
      n121 = Select(t=w206, s="PID Regler Speed Control\nWave Torque Reference", f=w261) -> (s? t:f=w262:dbl)
      n122 = Select(t=w252, s=w256, f=w251) -> (s? t:f=w257:dbl)
      n123 = xnode "Read/Write Control"("FPGA VI Reference In"=w225, "error in"=w311) -> ("FPGA VI Reference Out"=w384:refnum<k20>, "error out"=w310:errorcluster, "Mod5/Error Brake L"=w382:bool, "Mod5/Ready Brake L"=w381:bool, "Mod5/Temperature Brake L"=w380:bool, "Mod5/Alarm 1 Brake L"=w379:bool, "Mod5/Alarm 2 Brake L"=w378:bool, "Mod5/Error Brake R"=w377:bool, "Mod5/Ready Brake R"=w376:bool, "Mod5/Temperature Brake R"=w375:bool, "Mod5/Alarm 1 Brake R"=w374:bool, "Mod5/Alarm 2 Brake R"=w373:bool, "Mod6/Error Brake back"=w294:bool, "Mod6/Ready Brake back"=w293:bool, "Mod6/Temperature Brake back"=w292:bool, "Mod6/Alarm 1 Brake back"=w291:bool, "Mod6/Alarm 2 Brake back"=w290:bool)
      n124 = Bundle("Mod5/Error Brake L"=w382, "Mod5/Ready Brake L"=w381, "Mod5/Temperature Brake L"=w380, "Mod5/Alarm 1 Brake L"=w379, "Mod5/Alarm 2 Brake L"=w378, "Mod5/Error Brake R"=w377, "Mod5/Ready Brake R"=w376, "Mod5/Temperature Brake R"=w375, "Mod5/Alarm 1 Brake R"=w374, "Mod5/Alarm 2 Brake R"=w373) -> (→"Report L-R":T22)  [unwired: 1 in]
      n125 = Bundle("Mod6/Error Brake back"=w294, "Mod6/Ready Brake back"=w293, "Mod6/Temperature Brake back"=w292, "Mod6/Alarm 1 Brake back"=w291, "Mod6/Alarm 2 Brake back"=w290) -> (→"Report H":T23)  [unwired: 1 in]
      n126 = Divide(x="ACC_FeedFw", y=10.0) -> (x/y=w178:dbl)
      n127 = call-poly <vilib>:"PID Output Rate Limiter.vi"("output rate (EGU/min)"="output rate (EGU/min)", "initial output"=w178, "input (controller output)"=w178) -> ("output"=w197:dbl)  [unwired: 5 in, 1 out]
      n128 = case shown="\"L-R\"" w157 {
        frame "H" {
          w445 = 0.0
          w446 = FALSE ("Control_LR")
          n129 = local write "Torque_Reference_LR"(w445) -> ()
          n130 = local write "Speed_Reference_LR"(w445) -> ()
          n131 = local write "Brake_LR"(w446) -> ()
          n132 = local write "Control_LR"(w446) -> ()
        }
        frame "L-R" {
          w447 = 0.0
          w448 = FALSE ("Brake\nFrei H")
          n133 = local write "Speed \nReferance H"(w447) -> ()
          n134 = local write "Torque Reference H"(w447) -> ()
          n135 = local write "Brake_H"(w448) -> ()
          n136 = local write "Control_H"(w448) -> ()
        }
        frame "H-L-R" {
        }
        frame "System", Default {
        }
      }
      n137 = Select(t="Count (mSec) Ramp LR", s=w122, f="Count (mSec) Normal LR") -> (s? t:f=w267:u32)
      n138 = Select(t="Count (mSec) Ramp H", s=w194, f="Count (mSec) H") -> (s? t:f=w199:u32)
      n139 = case shown="0, Default" w146 {
        frame 0, Default {
          w452 = TRUE ("Ramp H Stop")
          w453 = FALSE
          w454 = 0.0
          w455 = FALSE ("Brake\nFrei H")
          n140 = local write "Ramp LR Stop"(w452) -> ()
          n141 = local write "Ramp H Stop"(w452) -> ()
          n142 = local write "Cruise Control Stop"(w452) -> ()
          n143 = local write "Control_LR"(w453) -> ()
          n144 = local write "Load Percent of Engine Speed"(w453) -> ()
          n145 = local write "Control_H"(w453) -> ()
          n146 = local write "PID Regler Speed Control\nWave Torque Reference"(w453) -> ()
          n147 = local write "Release Speed Control"(w453) -> ()
          n148 = local write "Speed_Reference_LR"(w454) -> ()
          n149 = local write "Speed Control Soll"(w454) -> ()
          n150 = local write "Torque_Reference_LR"(w454) -> ()
          n151 = local write "Torque Reference H"(w454) -> ()
          n152 = local write "Speed \nReferance H"(w454) -> ()
          n153 = local write "Brake_LR"(w455) -> ()
          n154 = local write "Brake_H"(w455) -> ()
        }
        frame 1 {
          w456 = FALSE
          n155 = local write "Release Speed Control"(w456) -> ()
          n156 = local write "PID Regler Speed Control\nWave Torque Reference"(w456) -> ()
        }
        frame 2 {
        }
      }
      n157 = Unbundle By Name("Spd_Cal_R") -> ("Gain"=w128:dbl, "Offset"=w126:dbl)
      n158 = Unbundle By Name("Spd_Cal_L") -> ("Gain"=w133:dbl, "Offset"=w130:dbl)
      n159 = Unbundle By Name("Tq_Cal_H") -> ("Gain_H"=w186:dbl, "Offset_H"=w183:dbl)
      n160 = Unbundle By Name("Spd_Cal_H") -> ("Gain"=w120:dbl, "Offset"=w108:dbl)
      n161 = Unbundle By Name("Tq_Cal_L") -> ("Gain"=w135:dbl, "Offset"=w136:dbl)
      n162 = Unbundle By Name("Tq_Cal_R") -> ("Gain"=w138:dbl, "Offset"=w137:dbl)
      n163 = feedback #2() -> (w209:dbl)  [unwired: 1 in]
      n164 = Add(x=w108, y=-100.0) -> (x+y=w109:dbl)
      n165 = Select(t=w108, s="Control_H", f=w109) -> (s? t:f=w112:dbl)
      n166 = feedback #3() -> (w168:dbl)  [unwired: 1 in]
      n167 = Select(t=w168, s=w205, f=w209) -> (s? t:f=w208:dbl)
      n168 = Select(t=w208, s="PID Regler Speed Control\nWave Torque Reference", f=w261) -> (s? t:f=w259:dbl)
      n169 = xnode "Read/Write Control"("FPGA VI Reference In"=w384, "error in"=w310, "Mod4/Clutch"="Clutch\nOpen", "Mod3/Speed Control Release"="Release Speed Control", "Speed Control Soll (%)"=w257, "Mod3/Engine Pre Glow ON"="Pre Glow\nOn", "Mod3/Start Engine"="Engine\nStart", "Mod3/Engine Ignition ON"="Ignition\nOn", "Mod3/Fuel Pump ON"="Fuel\nOn", "Mod4/Temperature Control OFF"="Temperature Control\nWait", "Mod4/Temperature Control Release"="Temperature Control \nRelease", "Regler Speed Control"="Release Speed Control", "Parameter Speed Control"=w262, "Ist Speed Control"=w259, "Count (mSec) Fahrhebel"="Count (mSec) Speed Control", "E-Acc_1"="E-Acc_1", "E-Acc_2"="E-Acc_2", "ACC_FeedFw"=w197, "FeedFw_Ena"="FeedFw_Ena") -> ("FPGA VI Reference Out"=w361:refnum<k20>, "error out"=w309:errorcluster, "Mod6/Clutch closed"=w217:bool, "Mod6/Clutch open"=w218:bool, "Speed_cmd"=w354:fxp<+/-,17,6>)  [unwired: 2 out]
      n170 = Bundle("Mod6/Clutch open"=w218, "Mod6/Clutch closed"=w217) -> (→"Clutch":T24)  [unwired: 1 in]
      n171 = Multiply(x=w354, y=10.0) -> (x*y=→"Speed Control":dbl)
      n172 = feedback #4() -> (w325:dbl)  [unwired: 1 in]
      n173 = xnode "Read/Write Control"("FPGA VI Reference In"=w361, "error in"=w309, "Mod3/Control ON Brake L"="Control_LR", "Mod3/Control Reset Brake L"="Reset_LR", "Mod3/Brake Performance ON Brake L"="Brake_LR", "Mod3/Unit ON Brake L"="Speed_Ref", "Mod3/Control ON Brake R"="Control_LR", "Mod3/Control Reset Brake R"="Reset_LR", "Mod3/Brake Performance ON Brake R"="Brake_LR", "Mod3/Unit ON Brake R"="Speed_Ref", "Mod4/Control ON Brake H"="Control_H", "Mod4/Control Reset Brake H"="Reset_H", "Mod4/Brake Performance ON Brake H"="Brake_H", "Mod4/Unit ON Brake H"="Speed_Ref_H", "Parameter Brake L"=w124, "Parameter Brake R"=w123, "Parameter Brake H"=w211, "Mod7/Out 1"=w325, "Engine Speed/moment LR"="Engine Speed/moment LR", "Count (mSec)"=w267, "Count (mSec) H"=w199, "Mod7/Out 2"=w168) -> ("FPGA VI Reference Out"=w279:refnum<k20>, "error out"=w308:errorcluster, "Mod2/Engine Speed Brake L"=w74:fxp<+/-,20,5>, "Mod2/Engine Speed Brake R"=w73:fxp<+/-,20,5>, "Mod8/Torque Brake L"=w72:fxp<+/-,24,5>, "Mod8/Torque Brake  R"=w71:fxp<+/-,24,5>, "Mod2/Engine Speed Brake H"=w70:fxp<+/-,20,5>, "Mod8/Torque Brake H"=w69:fxp<+/-,24,5>)
      n174 = Absolute Value(x=w70) -> (abs(x)=w296:fxp<+,20,5>)
      n175 = Absolute Value(x=w74) -> (abs(x)=w368:fxp<+,20,5>)
      n176 = Absolute Value(x=w73) -> (abs(x)=w369:fxp<+,20,5>)
      n177 = Negate(x=w71) -> (-x=w364:fxp<+/-,25,6>)
      n178 = Multiply(x=w133, y=w368) -> (x*y=w131:dbl)
      n179 = Multiply(x=w72, y=w135) -> (x*y=w144:dbl)
      n180 = Multiply(x=w296, y=w120) -> (x*y=w119:dbl)
      n181 = Multiply(x=w369, y=w128) -> (x*y=w127:dbl)
      n182 = Multiply(x=w69, y=w186) -> (x*y=w185:dbl)
      n183 = Multiply(x=w364, y=w138) -> (x*y=w141:dbl)
      n184 = Add(x=w127, y=w126) -> (x+y=w125:dbl)
      n185 = Add(x=w131, y=w130) -> (x+y=w132:dbl)
      n186 = Add(x=w144, y=w136) -> (x+y=w143:dbl)
      n187 = Add(x=w185, y=w183) -> (x+y=w184:dbl)
      n188 = Add(x=w141, y=w137) -> (x+y=w142:dbl)
      n189 = Add(x=w119, y=w112) -> (x+y=w118:dbl)
      n190 = Add(x=w143, y=w142) -> (x+y=w249:dbl)
      n191 = call <vilib>:"Mean PtByPt.vi"("x"=w132, "sample length"="sample length LR") -> ("mean"=w68:dbl)  [unwired: 2 in, 1 out]
      n192 = call <vilib>:"Mean PtByPt.vi"("x"=w142, "sample length"="sample length DM") -> ("mean"=w64:dbl)  [unwired: 2 in, 1 out]
      n193 = call <vilib>:"Mean PtByPt.vi"("x"=w125, "sample length"="sample length LR") -> ("mean"=w66:dbl)  [unwired: 2 in, 1 out]
      n194 = call <vilib>:"Mean PtByPt.vi"("x"=w143, "sample length"="sample length DM") -> ("mean"=w65:dbl)  [unwired: 2 in, 1 out]
      n195 = call <vilib>:"Mean PtByPt.vi"("x"=w118, "sample length"="sample length H") -> ("mean"=w62:dbl)  [unwired: 2 in, 1 out]
      n196 = call <vilib>:"Mean PtByPt.vi"("x"=w184, "sample length"="sample length H") -> ("mean"=w61:dbl)  [unwired: 2 in, 1 out]
      n197 = Divide(x=w61, y="Transmisssion H") -> (x/y=w172:dbl)
      n198 = Subtract(x=w68, y=w66) -> (x-y=w67:dbl)
      n199 = Add(x=w68, y=w66) -> (x+y=w366:dbl)
      n200 = Add(x=w65, y=w64) -> (x+y=w245:dbl)
      n201 = Add(x=w65, y=w64) -> (x+y=w304:dbl)
      n202 = call <vilib>:"Mean PtByPt.vi"("x"=w172, "sample length"="sample length H") -> ("mean"=w170:dbl)  [unwired: 2 in, 1 out]
      n203 = Multiply(x=w62, y="Transmisssion H") -> (x*y=→"Speed with Transmission H":dbl)
      n204 = Divide(x=w249, y="Transmission LR") -> (x/y=w247:dbl)
      n205 = Divide(x=w245, y="Transmission LR") -> (x/y=w222:dbl)
      n206 = Divide(x=w304, y="Transmission LR") -> (x/y=w231:dbl)
      n207 = call <vilib>:"Mean PtByPt.vi"("x"=w170, "sample length"="sample length H") -> ("mean"=w169:dbl)  [unwired: 2 in, 1 out]
      "Torque with Transmission  H" <- w169
      n208 = Build Array(w68, w67, w66, w65, w64, w62, w61) -> ()  [unwired: 1 out]
      n209 = Multiply(x=w222, y="Loss Factor") -> (x*y=w223:dbl)
      n210 = Multiply(x=w366, y=0.5) -> (x*y=w365:dbl)
      n211 = Subtract(x=w169, y=w183) -> (x-y=w182:dbl)
      n212 = Multiply(x=w231, y="Loss Factor") -> (x*y=→"Torque with Transmission":dbl)
      n213 = Divide(x=w247, y=200.0 ("Tq_cal")) -> (x/y=w258:dbl)
      n214 = feedback-in #2(w258) -> ()
      n215 = Divide(x=w182, y=w186) -> (x/y=w202:dbl)
      n216 = feedback-in #3(w202) -> ()
      n217 = Multiply(x=w365, y="Transmission LR") -> (x*y=→"Speed with Transmission":dbl)
      n218 = Divide(x=w223, y=400.0) -> (x/y=w324:dbl)
      n219 = Add(x=w324, y=5.0) -> (x+y=w244:dbl)
      n220 = call <vilib>:"Mean PtByPt.vi"("x"=w244, "sample length"="sample length DM") -> ("mean"=w243:dbl)  [unwired: 2 in, 1 out]
      n221 = feedback-in #4(w243) -> ()
    }
    n222 = while {
      stop <- w25 stop-if-true
      # "CHeck This"
      n223 = case shown="True" "Load Percent of Engine Speed" {
        frame False {
        }
        frame True {
          n224 = while {
            stop <- w36 stop-if-true
            n225 = local read "Load Percent of Engine Speed"() -> (w37:bool)
            n226 = shared-variable "NI-cRIO9082-AKZ1\\RT Library.lvlib\\Matrix"() -> (w29:dbl[][])  [unwired: 1 in, 1 out]
            n227 = local read "Speed with Transmission"() -> (w33:dbl)
            n228 = local read "Speed \nReferance H"() -> (w31:dbl)
            n229 = local read "Mod6/Unit H"() -> (w34:bool)
            n230 = Array Size(array=w29) -> (size(s)=w28:i32[])
            n231 = Not(x=w37) -> (.not. x?=w35:bool)
            n232 = Index Array(array=w28) -> (element=w27:i32)  [unwired: 1 in]
            n233 = local read "Stop"() -> (w38:bool)
            n234 = Select(t=w31, s=w34, f=w33) -> (s? t:f=w32:dbl)
            n235 = Decrement(x=w27) -> (x-1=w30:i32)
            n236 = Or(x=w38, y=w35) -> (x .or. y?=w36:bool)
            n237 = for {
              N: w30 -> [_]
              tunnel: w32 -> [w44]
              shift-right: [w42] -> _
              shift-left: w29 -> [w42]
              i -> [w41]
              n238 = Increment(x=w41) -> (x+1=w43:i32)
              n239 = Index Array(array=w42, index (row)=w41, index (col)=0 ("Index (Spalte)")) -> (element=w45:dbl)
              n240 = Index Array(array=w42, index (row)=w41, index (col)=1 ("Deaktivierter Index (Spalte)")) -> (element=w52:dbl)
              n241 = Index Array(array=w42, index (row)=w41, index (col)=2 ("disabled index (col)")) -> (element=w39:dbl)
              n242 = Greater Or Equal?(x=w44, y=w45) -> (x >= y?=w49:bool)
              n243 = Index Array(array=w42, index (row)=w43, index (col)=0 ("Index (Spalte)")) -> (element=w46:dbl)
              n244 = Less Or Equal?(x=w44, y=w46) -> (x <= y?=w48:bool)
              n245 = And(x=w49, y=w48) -> (x .and. y?=w47:bool)
              n246 = case shown="True" w47 {
                tunnel: w52 -> [_ w58]
                tunnel: w39 -> [_ w54]
                frame False {
                }
                frame True {
                  n247 = local write "ACC_FeedFw"(w54) -> ()
                  n248 = local read "Mod6/Unit H"() -> (w56:bool)
                  n249 = Multiply(x="Percent", y=w58) -> (x*y=w55:dbl)
                  n250 = case shown="False" w56 {
                    tunnel: w55 -> [w59 w60]
                    frame False {
                      n251 = local write "Torque_Reference_LR"(w59) -> ()
                    }
                    frame True {
                      n252 = local write "Torque Reference H"(w60) -> ()
                    }
                  }
                }
              }
            }
          }
        }
      }
      n253 = local read "Stop"() -> (w25:bool)
    }
    n254 = xnode "Invoke Method"("FPGA VI Reference In"=w23, "error in"=w21) -> ("FPGA VI Reference Out"=w15:refnum<k20>, "error out"=w14:errorcluster)
    n255 = xnode "Close FPGA VI Reference"("FPGA VI Reference In"=w15, "error in"=w14) -> ()  [unwired: 1 out]
  }
  n256 = while {
    shift-right: [w467] -> _
    shift-left: string[] ["Initialize"] -> [w466]
    shift-right: [w458] -> _
    shift-left: T15 {"Ramp Pattern"=[], "Ramp Type"=0, "Ramp Step"=0, "Ramp Start H"=0.0, "Ramp End  H"=0.0, "No of Ramps"=60, "Loop Time"=100, "LR Timer Done"=FALSE, "LR Ramp On"=FALSE, "Ramp Time Target"=100} -> [w460]
    shift-right: [w461] -> _
    shift-left: errorcluster {"status"=FALSE, "code"=0, "source"=""} ("error constant") -> [w462]
    tunnel: string[] ["Ramp H Start", "Start H Ramp Down"] -> [w459]
    stop <- "stop 3" stop-if-true
    # "H Speed Control"
    n257 = Delete From Array(array=w466, index=0) -> (deleted portion=w464:string, array with subset deleted=w463:string[])  [unwired: 1 in]
    n258 = case shown="\"Poll\", Default" w464 {
      tunnel: [w471 w475 w491 w519 w535 w547 w575] -> w467
      tunnel: w463 -> [w471 w476 w504 w520 w544 w559 w575]
      tunnel: w462 -> [w470 w479 w495 w517 w543 w558 w574]
      tunnel: [w470 w479 w495 w517 w543 w558 w574] -> w461
      tunnel: w460 -> [w469 w474 w498 w515 w538 w550 w573]
      tunnel: [w469 w474 w497 w516 w536 w549 w572] -> w458
      tunnel: w459 -> [_ w478 _ _ _ _ _]
      frame "Initialize" {
      }
      frame "Poll", Default {
        n259 = Build Array("Ramp H Start", "Ramp H Down") -> (w477:bool[])
        n260 = call "Add triggered Events.vi"("Triggers"=w477, "States  List"=w478, "List In"=w476) -> ("List Out"=w475:string[])  [unwired: 8 in]
      }
      frame "Ramp H Start" {
        w502 = 800.0
        n261 = local read "Transmisssion H"() -> (w487:dbl)
        n262 = Divide(x="End Ramp H", y=w487) -> (x/y=w501:dbl)
        n263 = Divide(x="Start Ramp H", y=w487) -> (x/y=w500:dbl)
        n264 = Select(t=w501, s="Transmission with H", f="End Ramp H") -> (s? t:f=w499:dbl)
        n265 = Select(t=w500, s="Transmission with H", f="Start Ramp H") -> (s? t:f=w484:dbl)
        "Startwert Ramp H" <- w484
        n266 = local write "Ramp H Activ"(TRUE) -> ()
        n267 = Divide(x=w499, y=w502) -> (x/y=w494:dbl)
        n268 = Divide(x=w484, y=w502) -> (x/y=w493:dbl)
        n269 = Multiply(x="Time (Sec) Ramp H", y=100) -> (x*y=w492:i32)
        n270 = Build Array (concatenate)(w504, "H Ramp Up") -> (w491:string[])
        n271 = call-poly <vilib>:"Ramp Pattern.vi"("type"="type Ramp H", "start"=w493, "end"=w494, "samples"=w492) -> ("Ramp Pattern"=w496:dbl[])  [unwired: 6 in, 1 out]
        n272 = Bundle By Name(cluster=w498, "No of Ramps"=w492, "Ramp End  H"=w494, "Ramp Start H"=w493, "Ramp Pattern"=w496, "Ramp Type"="type Ramp H", "Loop Time"="milliseconds to wait Ramp H", "LR Ramp On"=TRUE) -> (w497:T15)
      }
      frame "H Ramp Up" {
        n273 = Unbundle By Name(w515) -> ("Ramp Pattern"=w510:dbl[], "Ramp Step"=w508:i32)
        n274 = local read "Ramp H Stop"() -> (w506:bool)
        n275 = Array Size(array=w510) -> (size(s)=w509:i32)
        n276 = Subtract(x=w509, y=1) -> (x-y=w513:i32)
        n277 = Less Or Equal?(x=w513, y=w508) -> (x <= y?=w512:bool)
        n278 = Or(x=w506, y=w512) -> (x .or. y?=w511:bool)
        n279 = Index Array(array=w510, index=w508) -> (element=w505:dbl)
        n280 = case shown="True" w511 {
          tunnel: [w521 _] -> w518
          tunnel: w515 -> [w525 w531]
          tunnel: [w524 w530] -> w516
          tunnel: w505 -> [_ w529]
          tunnel: w508 -> [w523 _]
          tunnel: string[] ["Poll", "H Ramp Up"] -> [w521 _]
          frame False {
            n281 = Increment(x=w523) -> (x+1=w522:i32)
            n282 = Bundle By Name(cluster=w525, "Ramp Step"=w522) -> (w524:T15)
          }
          frame True {
            n283 = local write "Ramp H  LED"(TRUE ("Ramp H  LED")) -> ()
            n284 = Bundle By Name(cluster=w531, "Ramp End  H"=w529, "Ramp Step"=0, "LR Ramp On"=FALSE) -> (w530:T15)
          }
        }
        n285 = local write "Output Ramp H"(w505) -> ()
        n286 = Build Array (concatenate)(w520, w518) -> (w519:string[])
      }
      frame "Start H Ramp Down" {
        n287 = Unbundle By Name(w538) -> ("No of Ramps"=w540:i32, "Ramp Start H"=w542:dbl, "Ramp End  H"=w541:dbl, "Ramp Type"=w539:u16)
        n288 = local write "Ramp LR  LED"(FALSE ("Ramp LR  LED")) -> ()
        n289 = call-poly <vilib>:"Ramp Pattern.vi"("type"=w539, "start"=w541, "end"=w542, "samples"=w540) -> ("Ramp Pattern"=w537:dbl[])  [unwired: 6 in, 1 out]
        n290 = Bundle By Name(cluster=w538, "LR Ramp On"=TRUE, "Ramp Pattern"=w537) -> (w536:T15)
        n291 = Build Array (concatenate)(w544, "H RampDown") -> (w535:string[])
      }
      frame "H RampDown" {
        n292 = Unbundle By Name(w550) -> ("Ramp Step"=w548:i32, "Ramp Pattern"=w553:dbl[])
        n293 = Array Size(array=w553) -> (size(s)=w552:i32)
        n294 = Subtract(x=w552, y=1) -> (x-y=w555:i32)
        n295 = Equal?(x=w555, y=w548) -> (x = y?=w556:bool)
        n296 = local read "Ramp LR Stop"() -> (w557:bool)
        n297 = Index Array(array=w553, index=w548) -> (element=w545:dbl)
        n298 = local write "Output Ramp H"(w545) -> ()
        n299 = Or(x=w556, y=w557) -> (x .or. y?=w551:bool)
        n300 = case shown="False" w551 {
          tunnel: w550 -> [w564 w569]
          tunnel: [w563 w567] -> w549
          tunnel: w548 -> [w562 _]
          tunnel: ["LR RampDvown" "H Ramp End"] -> w546
          frame False {
            n301 = Increment(x=w562) -> (x+1=w561:i32)
            n302 = Bundle By Name(cluster=w564, "Ramp Step"=w561) -> (w563:T15)
          }
          frame True {
            n303 = Bundle By Name(cluster=w569, "LR Ramp On"=FALSE, "Ramp Step"=0) -> (w567:T15)
          }
        }
        n304 = Build Array (concatenate)(w559, w546) -> (w547:string[])
      }
      frame "H Ramp End" {
        w570 = FALSE
        n305 = local write "Ramp H  LED"(w570) -> ()
        n306 = local write "Ramp H Start"(w570) -> ()
        n307 = local write "Ramp H Activ"(w570) -> ()
        n308 = local write "Ramp H Stop"(w570) -> ()
        n309 = Bundle By Name(cluster=w573, "Loop Time"=u32 100) -> (w572:T15)
      }
    }
    n310 = Unbundle By Name(w458) -> ("Loop Time"=w457:u32)
    n311 = call "Wait Until Next Multiple2"("Count(mSec)"=w457) -> ()  [unwired: 1 out]
  }
  n312 = while {
    shift-right: [w586] -> _
    shift-left: string[] ["Initialize"] -> [w585]
    shift-right: [w577] -> _
    shift-left: T16 {"FPGA VI Ref"=refnum, "Ramp Pattern"=[], "Ramp Type"=0, "Ramp Step"=0, "Ramp Start LR"=0.0, "Ramp End  LR"=0.0, "No of Ramps"=60, "Loop Time"=100, "LR Timer Done"=FALSE, "LR Ramp On"=FALSE, "Ramp Time Target"=100} -> [w579]
    shift-right: [w580] -> _
    shift-left: errorcluster {"status"=FALSE, "code"=0, "source"=""} ("error constant") -> [w581]
    tunnel: string[] ["Ramp Lr Start", "Start LR Ramp Down"] -> [w578]
    stop <- "stop 2" stop-if-true
    # "LR Speed Control"
    n313 = Delete From Array(array=w585, index=0) -> (deleted portion=w583:string, array with subset deleted=w582:string[])  [unwired: 1 in]
    n314 = case shown="\"Poll\", Default" w583 {
      tunnel: [w590 w593 w602 w613 w642 w658 w669 w698] -> w586
      tunnel: w582 -> [w590 w594 w602 w627 w643 w667 w682 w698]
      tunnel: w581 -> [w589 w599 w601 w617 w640 w666 w681 w696]
      tunnel: [w589 w598 w601 w617 w640 w666 w681 w696] -> w580
      tunnel: w579 -> [w588 w591 w600 w620 w638 w661 w672 w695]
      tunnel: [w588 w591 w600 w619 w639 w659 w671 w694] -> w577
      tunnel: w578 -> [_ w597 _ _ _ _ _ _]
      frame "Initialize" {
      }
      frame "Poll", Default {
        n315 = shared-variable "NI-cRIO9082-AKZ1\\RT Library.lvlib\\Ramp LR Start"(error in=w599) -> (w596:bool, error out=w598:errorcluster)
        n316 = Build Array(w596, "Ramp LR Down") -> (w595:bool[])
        n317 = call "Add triggered Events.vi"("Triggers"=w595, "States  List"=w597, "List In"=w594) -> ("List Out"=w593:string[])  [unwired: 8 in]
      }
      frame "Open FPGA Reference" {
      }
      frame "Ramp Lr Start" {
        w625 = 300.0
        n318 = local read "Transmission LR"() -> (w622:dbl)
        n319 = Divide(x="End Ramp LR", y=w622) -> (x/y=w624:dbl)
        n320 = Divide(x="Start Ramp LR", y=w622) -> (x/y=w623:dbl)
        n321 = local write "Ramp LR active"(TRUE) -> ()
        n322 = Select(t=w624, s="Transmission LR\nwith", f="End Ramp LR") -> (s? t:f=w621:dbl)
        n323 = Select(t=w623, s="Transmission LR\nwith", f="Start Ramp LR") -> (s? t:f=w608:dbl)
        "Startwert Ramp LR" <- w608
        n324 = Divide(x=w621, y=w625) -> (x/y=w616:dbl)
        n325 = Divide(x=w608, y=w625) -> (x/y=w615:dbl)
        n326 = Multiply(x="Time (Sec) Ramp LR", y=100) -> (x*y=w614:i32)
        n327 = Build Array (concatenate)(w627, "LR Ramp Up") -> (w613:string[])
        n328 = call-poly <vilib>:"Ramp Pattern.vi"("type"="type Ramp LR", "start"=w615, "end"=w616, "samples"=w614) -> ("Ramp Pattern"=w618:dbl[])  [unwired: 6 in, 1 out]
        n329 = Bundle By Name(cluster=w620, "No of Ramps"=w614, "Ramp End  LR"=w616, "Ramp Start LR"=w615, "Ramp Pattern"=w618, "Ramp Type"="type Ramp LR", "Loop Time"="milliseconds to wait Ramp LR", "LR Ramp On"=TRUE) -> (w619:T16)
      }
      frame "LR Ramp Up" {
        n330 = Unbundle By Name(w638) -> ("Ramp Pattern"=w632:dbl[], "Ramp Step"=w629:i32)
        n331 = local read "Ramp LR Stop"() -> (w634:bool)
        n332 = Array Size(array=w632) -> (size(s)=w631:i32)
        n333 = Subtract(x=w631, y=1) -> (x-y=w636:i32)
        n334 = Less Or Equal?(x=w636, y=w629) -> (x <= y?=w635:bool)
        n335 = Or(x=w634, y=w635) -> (x .or. y?=w633:bool)
        n336 = Index Array(array=w632, index=w629) -> (element=w630:dbl)
        n337 = case shown="False" w633 {
          tunnel: [w644 _] -> w641
          tunnel: w638 -> [w648 w654]
          tunnel: [w647 w653] -> w639
          tunnel: w630 -> [_ w652]
          tunnel: w629 -> [w646 _]
          tunnel: string[] ["Poll", "LR Ramp Up"] -> [w644 _]
          frame False {
            n338 = Increment(x=w646) -> (x+1=w645:i32)
            n339 = Bundle By Name(cluster=w648, "Ramp Step"=w645) -> (w647:T16)
          }
          frame True {
            n340 = Bundle By Name(cluster=w654, "Ramp End  LR"=w652, "Ramp Step"=0, "LR Ramp On"=FALSE) -> (w653:T16)
            n341 = local write "Ramp LR  LED"(TRUE ("Ramp LR  LED")) -> ()
          }
        }
        n342 = local write "Output Ramp LR"(w630) -> ()
        n343 = Build Array (concatenate)(w643, w641) -> (w642:string[])
      }
      frame "Start LR Ramp Down" {
        n344 = Unbundle By Name(w661) -> ("No of Ramps"=w663:i32, "Ramp Start LR"=w665:dbl, "Ramp End  LR"=w664:dbl, "Ramp Type"=w662:u16)
        n345 = local write "Ramp LR  LED"(FALSE ("Ramp LR  LED")) -> ()
        n346 = call-poly <vilib>:"Ramp Pattern.vi"("type"=w662, "start"=w664, "end"=w665, "samples"=w663) -> ("Ramp Pattern"=w660:dbl[])  [unwired: 6 in, 1 out]
        n347 = Bundle By Name(cluster=w661, "LR Ramp On"=TRUE, "Ramp Pattern"=w660) -> (w659:T16)
        n348 = Build Array (concatenate)(w667, "LR RampDown") -> (w658:string[])
      }
      frame "LR RampDown" {
        n349 = Unbundle By Name(w672) -> ("Ramp Step"=w670:i32, "Ramp Pattern"=w675:dbl[])
        n350 = Array Size(array=w675) -> (size(s)=w674:i32)
        n351 = Subtract(x=w674, y=1) -> (x-y=w677:i32)
        n352 = Equal?(x=w677, y=w670) -> (x = y?=w678:bool)
        n353 = local read "Ramp LR Stop"() -> (w679:bool)
        n354 = Index Array(array=w675, index=w670) -> (element=w680:dbl)
        n355 = local write "Output Ramp LR"(w680) -> ()
        n356 = Or(x=w678, y=w679) -> (x .or. y?=w673:bool)
        n357 = case shown="True" w673 {
          tunnel: w672 -> [w687 w692]
          tunnel: [w686 w690] -> w671
          tunnel: w670 -> [w685 _]
          tunnel: ["LR RampDown" "LR Ramp End"] -> w668
          frame False {
            n358 = Increment(x=w685) -> (x+1=w684:i32)
            n359 = Bundle By Name(cluster=w687, "Ramp Step"=w684) -> (w686:T16)
          }
          frame True {
            n360 = Bundle By Name(cluster=w692, "LR Ramp On"=FALSE, "Ramp Step"=0) -> (w690:T16)
          }
        }
        n361 = Build Array (concatenate)(w682, w668) -> (w669:string[])
      }
      frame "LR Ramp End" {
        w697 = FALSE
        n362 = local write "Ramp LR active"(w697) -> ()
        n363 = local write "Ramp LR Stop"(w697) -> ()
        n364 = local write "Ramp LR Start"(w697) -> ()
        n365 = Bundle By Name(cluster=w695, "Loop Time"=u32 100) -> (w694:T16)
      }
    }
    n366 = Unbundle By Name(w577) -> ("Loop Time"=w576:u32)
    n367 = call "Wait Until Next Multiple"("Count(mSec)"=w576) -> ()  [unwired: 1 out]
  }
  n368 = while {
    shift-right: [w709] -> _
    shift-left: string[] ["Initialize"] -> [w708]
    shift-right: [w700] -> _
    shift-left: T14 {"Ramp Pattern"=[], "Ramp Type"=0, "Ramp Step"=0, "Ramp Start Cruise"=0.0, "Ramp End  Cruise"=0.0, "No of Ramps"=60, "Loop Time"=100, "LR Timer Done"=FALSE, "LR Ramp On"=FALSE, "Ramp Time Target"=100} -> [w702]
    shift-right: [w703] -> _
    shift-left: errorcluster {"status"=FALSE, "code"=0, "source"=""} ("error constant") -> [w704]
    tunnel: string[] ["Ramp Cruise Start", "Start Cruise Ramp Down"] -> [w701]
    stop <- "stop 4" stop-if-true
    # "Cruise Control"
    n369 = Delete From Array(array=w708, index=0) -> (deleted portion=w706:string, array with subset deleted=w705:string[])  [unwired: 1 in]
    n370 = case shown="\"Poll\", Default" w706 {
      tunnel: [w713 w717 w732 w756 w772 w785 w812] -> w709
      tunnel: w705 -> [w713 w718 w741 w757 w781 w796 w812]
      tunnel: w704 -> [w712 w721 w734 w754 w780 w795 w811]
      tunnel: [w712 w721 w734 w754 w780 w795 w811] -> w703
      tunnel: w702 -> [w711 w716 w737 w752 w775 w788 w810]
      tunnel: [w711 w716 w736 w753 w773 w787 w809] -> w700
      tunnel: w701 -> [_ w720 _ _ _ _ _]
      frame "Initialize" {
      }
      frame "Poll", Default {
        n371 = Build Array("Cruise Control Start", "Cruise Control Down") -> (w719:bool[])
        n372 = call "Add triggered Events.vi"("Triggers"=w719, "States  List"=w720, "List In"=w718) -> ("List Out"=w717:string[])  [unwired: 8 in]
      }
      frame "Ramp Cruise Start" {
        w725 = 10.0
        n373 = Divide(x="End Cruise Control", y=w725) -> (x/y=w739:dbl)
        n374 = Divide(x="Start Cruise Control", y=w725) -> (x/y=w738:dbl)
        "Startwert Ramp H 2" <- w738
        n375 = local write "Ramp Cruise Control  LED"(FALSE) -> ()
        n376 = local write "Cruise Control Aktive"(TRUE) -> ()
        n377 = Multiply(x="Time (Sec) Speed Control", y=100) -> (x*y=w733:i32)
        n378 = Build Array (concatenate)(w741, "Cruise Ramp Up") -> (w732:string[])
        n379 = call-poly <vilib>:"Ramp Pattern.vi"("type"="type Speed Control", "start"=w738, "end"=w739, "samples"=w733) -> ("Ramp Pattern"=w735:dbl[])  [unwired: 6 in, 1 out]
        n380 = Bundle By Name(cluster=w737, "No of Ramps"=w733, "Ramp End  Cruise"=w739, "Ramp Start Cruise"=w738, "Ramp Pattern"=w735, "Ramp Type"="type Speed Control", "Loop Time"="milliseconds to wait Speed Control", "LR Ramp On"=TRUE) -> (w736:T14)
      }
      frame "Cruise Ramp Up" {
        n381 = Unbundle By Name(w752) -> ("Ramp Pattern"=w747:dbl[], "Ramp Step"=w745:i32)
        n382 = local read "Cruise Control Stop"() -> (w742:bool)
        n383 = Array Size(array=w747) -> (size(s)=w746:i32)
        n384 = Subtract(x=w746, y=1) -> (x-y=w750:i32)
        n385 = Less Or Equal?(x=w750, y=w745) -> (x <= y?=w749:bool)
        n386 = Or(x=w742, y=w749) -> (x .or. y?=w748:bool)
        n387 = Index Array(array=w747, index=w745) -> (element=w743:dbl)
        n388 = case shown="True" w748 {
          tunnel: [w758 _] -> w755
          tunnel: w752 -> [w762 w768]
          tunnel: [w761 w767] -> w753
          tunnel: w743 -> [_ w766]
          tunnel: w745 -> [w760 _]
          tunnel: string[] ["Poll", "Cruise Ramp Up"] -> [w758 _]
          frame False {
            n389 = Increment(x=w760) -> (x+1=w759:i32)
            n390 = Bundle By Name(cluster=w762, "Ramp Step"=w759) -> (w761:T14)
          }
          frame True {
            n391 = local write "Ramp Cruise Control  LED"(TRUE) -> ()
            n392 = Bundle By Name(cluster=w768, "Ramp End  Cruise"=w766, "Ramp Step"=0, "LR Ramp On"=FALSE) -> (w767:T14)
          }
        }
        n393 = local write "Output Speed Control"(w743) -> ()
        n394 = Build Array (concatenate)(w757, w755) -> (w756:string[])
      }
      frame "Start Cruise Ramp Down" {
        n395 = Unbundle By Name(w775) -> ("No of Ramps"=w777:i32, "Ramp Start Cruise"=w779:dbl, "Ramp End  Cruise"=w778:dbl, "Ramp Type"=w776:u16)
        n396 = local write "Ramp Cruise Control  LED"(FALSE) -> ()
        n397 = call-poly <vilib>:"Ramp Pattern.vi"("type"=w776, "start"=w778, "end"=w779, "samples"=w777) -> ("Ramp Pattern"=w774:dbl[])  [unwired: 6 in, 1 out]
        n398 = Bundle By Name(cluster=w775, "LR Ramp On"=TRUE, "Ramp Pattern"=w774) -> (w773:T14)
        n399 = Build Array (concatenate)(w781, "Cruise RampDown") -> (w772:string[])
      }
      frame "Cruise RampDown" {
        n400 = Unbundle By Name(w788) -> ("Ramp Step"=w786:i32, "Ramp Pattern"=w791:dbl[])
        n401 = Array Size(array=w791) -> (size(s)=w790:i32)
        n402 = Subtract(x=w790, y=1) -> (x-y=w793:i32)
        n403 = Equal?(x=w793, y=w786) -> (x = y?=w794:bool)
        n404 = local read "Cruise Control Stop"() -> (w783:bool)
        n405 = Index Array(array=w791, index=w786) -> (element=w782:dbl)
        n406 = local write "Output Speed Control"(w782) -> ()
        n407 = Or(x=w794, y=w783) -> (x .or. y?=w789:bool)
        n408 = case shown="False" w789 {
          tunnel: w788 -> [w801 w806]
          tunnel: [w800 w804] -> w787
          tunnel: w786 -> [w799 _]
          tunnel: ["Cruise RampDown" "Cruise Ramp End"] -> w784
          frame False {
            n409 = Increment(x=w799) -> (x+1=w798:i32)
            n410 = Bundle By Name(cluster=w801, "Ramp Step"=w798) -> (w800:T14)
          }
          frame True {
            n411 = Bundle By Name(cluster=w806, "LR Ramp On"=FALSE, "Ramp Step"=0) -> (w804:T14)
          }
        }
        n412 = Build Array (concatenate)(w796, w784) -> (w785:string[])
      }
      frame "Cruise Ramp End" {
        w807 = FALSE
        n413 = local write "Cruise Control Stop"(w807) -> ()
        n414 = local write "Cruise Control Aktive"(w807) -> ()
        n415 = local write "Cruise Control Start"(w807) -> ()
        n416 = Bundle By Name(cluster=w810, "Loop Time"=u32 100) -> (w809:T14)
      }
    }
    n417 = Unbundle By Name(w700) -> ("Loop Time"=w699:u32)
    n418 = call "Wait Until Next Multiple3"("Count(mSec)"=w699) -> ()  [unwired: 1 out]
  }
